vi "HDF5_Write_Noise_Record.vi"(6 "RedundantFileNumber":i32, 7 "LogClust":T1={"base path"=path "C:/Users/Bruce Wayne/Desktop/SourceCode_20171218/thresholds.csv", "PathNow1"=path "", "PathNow2"=path "", "DateNow"="", "NAS path"=path "C:/Users/Bruce Wayne/Desktop/SourceCode_20171218/thresholds.csv", "LogFiltStage"=FALSE, "LogNoise_df_1"=FALSE, "LogNoise_df_2"=FALSE, "LogNoise_df_3"=FALSE, "LogNoise_df_4"=FALSE, "Config"={"UsrCfg"={"Paths"={"CfgFile"=path "", "LogFolder"=path "", "LogFile"=path "", "NAS path"=path "", "ThreshFile"=path "", "RedunFolder"=path ""}, "SampleRate"=12500.0}, "FP_User"={"#NoiseSums"=1, "Max_df"=1, "AvgAvg"=FALSE, "#Avg"=1, "AutoCenter"=FALSE, "Inclin"={"Vmin"=0.0, "Vmax"=0.0, "Angle_min"=0.0, "Angle_max"=0.0, "Offset"=0.0, "Pos_Neg"=FALSE}, "1"={"Cal_"={"Fine"=0.000213623046875, "Coarse_"=4194303.0}, "Beac"={"Fine"=4194303.0, "Coarse_"=1.0}, "Scale"={"Step4"=10000.0, "Step5"=4194303.0, "Step6"=1.0, "Step7"=10000.0}, "Offset"=0.0, "Scale_Noise"=4194303.0, "Scale_Step1"=65535.0, "Scale_In_RT"=1.0, "ScaleMeas"=0.999969482421875, "FreqsToRemove"=[0, 1633], "Width"=[0, 1633], "ScaleMeasEnum"=enum."50", "FilterEnab"=enum."Step 1"}, "2"={"Cal_"={"Fine"=0.000213623046875, "Coarse_"=4194303.0}, "Beac"={"Fine"=0.000213623046875, "Coarse_"=4194303.0}, "Scale"={"Step4"=0.0, "Step5"=4194303.0, "Step6"=1.0, "Step7"=10000.0}, "Offset"=0.0, "Scale_Noise"=4194303.0, "Scale_Step1"=65535.0, "Scale_In_RT"=1.0, "ScaleMeas"=0.999969482421875, "FreqsToRemove"=[0, 1633], "Width"=[0, 1633], "ScaleMeasEnum"=enum."50", "FilterEnab"=enum."Step 1"}, "3"={"Cal_"={"Fine"=0.000213623046875, "Coarse_"=4194303.0}, "Beac"={"Fine"=0.000213623046875, "Coarse_"=4194303.0}, "Scale"={"Step4"=0.0, "Step5"=4194303.0, "Step6"=1.0, "Step7"=10000.0}, "Offset"=0.0, "Scale_Noise"=4194303.0, "Scale_Step1"=65535.0, "Scale_In_RT"=1.0, "ScaleMeas"=0.999969482421875, "FreqsToRemove"=[0, 1633], "Width"=[0, 1633], "ScaleMeasEnum"=enum."50", "FilterEnab"=enum."Step 1"}, "4"={"Cal_"={"Fine"=0.000213623046875, "Coarse_"=4194303.0}, "Beac"={"Fine"=0.000213623046875, "Coarse_"=4194303.0}, "Scale"={"Step4"=0.0, "Step5"=4194303.0, "Step6"=1.0, "Step7"=10000.0}, "Offset"=0.0, "Scale_Noise"=4194303.0, "Scale_Step1"=1.0, "Scale_In_RT"=10000.0, "ScaleMeas"=0.999969482421875, "FreqsToRemove"=[0, 1633], "Width"=[0, 1633], "ScaleMeasEnum"=enum."50", "FilterEnab"=enum."Step 1"}, "Target to Probe"=enum."4", "SNR_Thresh"=1.0, "Paths"={"CfgFile"=path "", "LogFolder"=path "", "LogFile"=path "", "NAS path"=path "", "ThreshFile"=path "", "RedunFolder"=path ""}, "Connex_Location"="", "SimulateFPGA"=FALSE, "Deadband"=0.0}}, "HDFRefs1"={"File"=0, "ToneRefs"=[], "NoiseRefs"=[], "TC_Refs"={"Group_ref"=0, "TimeString_dset"=0, "TimeStamp_dset"=0, "TC0_LP1_Hi"=0, "TC1_LP1_MidHi"=0, "TC2_LP1_Mid"=0, "TC3_LP1_LoMid"=0, "TC4_LP1_Lo"=0, "TC5_LP2_Hi"=0, "TC6_LP2_MidHi"=0, "TC7_LP2_Mid"=0, "TC8_LP2_LoMid"=0, "TC9_LP2_Lo"=0, "TC10_HVAC_Cond_In"=0, "TC11_HVAC_Cond_Out"=0, "TC12_Gen_Exhaust"=0, "TC13_Tamb_Inter"=0}, "ValidRefs"={"Group_ref"=0, "Weath_Valid_dset"=0, "Disdr_Valid_dset"=0, "Saturat_dset"=0, "Alarm_Valid_dset"=0, "Time_Valid_dset"=0, "Time_AlarmChange_dset"=0, "Alarm_Source_dset"=0}, "DisdromRefs"={"BasicGroup_ref"=0, "TimeStamp_dset"=0, "TotalRainRate_dset"=0, "Liquid_dset"=0, "Solid_dset"=0, "TotalRain_dset"=0, "Visibility_dset"=0, "RadarReflect_dset"=0, "MaxDiam_dset"=0, "MeasdParticles_dset"=0, "ParticlMinSpeed_dset"=0, "ParticlMaxSpeed_dset"=0, "ParticlMinDiam_dset"=0, "NonHydrParticls_dset"=0, "NonHydrVolum_dset"=0, "UnknownParticls_dset"=0, "UnknownVolum_dset"=0, "HydromType_dset"=0, "SpectGroup_ref"=0, "Spectrum_dset"=0, "Status_dset_deprecated"=0}, "TE_Refs"={"Group_ref"=0, "TE_Temp1_dset"=0, "TE_Outp1_dset"=0, "TE_Temp2_dset"=0, "TE_Outp2_dset"=0, "TE_Temp3_dset"=0, "TE_Outp3_dset"=0, "TimeStamp"=0}, "UPS_Refs_Deprecated"={"Group_ref"=0, "TimeString_dset"=0, "TimeStamp_dset"=0, "V_dset"=0, "A_dset"=0, "Hz_dset"=0, "W_dset"=0, "%_dset"=0}, "Weath_Refs"={"Group_ref"=0, "TimeString_dset"=0, "TimeStamp_dset "=0, "WindSpd_dset"=0, "WindGusts_dset"=0, "WindDir_dset"=0, "WindDirSTD_dset"=0, "Temp_dset"=0, "Humidity_dset"=0, "Pressure_dset"=0, "RainRate_dset"=0, "RainFall_dset"=0}, "AI_Refs"={"Group_ref"=0, "TimeString_dset"=0, "TimeStamp_dset"=0, "AI0_dset"=0, "AI1_dset"=0, "AI2_dset"=0, "AI3_dset"=0, "AI4_dset"=0, "AI5_dset"=0, "AI6_dset"=0, "AI16_dset"=0, "AI17_dset"=0, "AI18_dset"=0, "AzStdDev_dset"=0, "AI19_dset"=0, "ElStdDev_dset"=0, "BlowerPwr_dset"=0}, "Filter_Refs"={"Filter_Group_ref"=0, "TimeStamp_dset"=0, "Filter_dset"=0}, "ADAM_Refs"={"Group_ref"=0, "ADAM_CoPol_dset"=0, "ADAM_XPol_dset"=0, "ADAM_Noise_dset"=0, "ADAM_CalBox_dset"=0, "TimeStamp"=0}, "Complex"=[]}, "HDFRefs2"={"File"=0, "ToneRefs"=[], "NoiseRefs"=[], "TC_Refs"={"Group_ref"=0, "TimeString_dset"=0, "TimeStamp_dset"=0, "TC0_LP1_Hi"=0, "TC1_LP1_MidHi"=0, "TC2_LP1_Mid"=0, "TC3_LP1_LoMid"=0, "TC4_LP1_Lo"=0, "TC5_LP2_Hi"=0, "TC6_LP2_MidHi"=0, "TC7_LP2_Mid"=0, "TC8_LP2_LoMid"=0, "TC9_LP2_Lo"=0, "TC10_HVAC_Cond_In"=0, "TC11_HVAC_Cond_Out"=0, "TC12_Gen_Exhaust"=0, "TC13_Tamb_Inter"=0}, "ValidRefs"={"Group_ref"=0, "Weath_Valid_dset"=0, "Disdr_Valid_dset"=0, "Saturat_dset"=0, "Alarm_Valid_dset"=0, "Time_Valid_dset"=0, "Time_AlarmChange_dset"=0, "Alarm_Source_dset"=0}, "DisdromRefs"={"BasicGroup_ref"=0, "TimeStamp_dset"=0, "TotalRainRate_dset"=0, "Liquid_dset"=0, "Solid_dset"=0, "TotalRain_dset"=0, "Visibility_dset"=0, "RadarReflect_dset"=0, "MaxDiam_dset"=0, "MeasdParticles_dset"=0, "ParticlMinSpeed_dset"=0, "ParticlMaxSpeed_dset"=0, "ParticlMinDiam_dset"=0, "NonHydrParticls_dset"=0, "NonHydrVolum_dset"=0, "UnknownParticls_dset"=0, "UnknownVolum_dset"=0, "HydromType_dset"=0, "SpectGroup_ref"=0, "Spectrum_dset"=0, "Status_dset_deprecated"=0}, "TE_Refs"={"Group_ref"=0, "TE_Temp1_dset"=0, "TE_Outp1_dset"=0, "TE_Temp2_dset"=0, "TE_Outp2_dset"=0, "TE_Temp3_dset"=0, "TE_Outp3_dset"=0, "TimeStamp"=0}, "UPS_Refs_Deprecated"={"Group_ref"=0, "TimeString_dset"=0, "TimeStamp_dset"=0, "V_dset"=0, "A_dset"=0, "Hz_dset"=0, "W_dset"=0, "%_dset"=0}, "Weath_Refs"={"Group_ref"=0, "TimeString_dset"=0, "TimeStamp_dset "=0, "WindSpd_dset"=0, "WindGusts_dset"=0, "WindDir_dset"=0, "WindDirSTD_dset"=0, "Temp_dset"=0, "Humidity_dset"=0, "Pressure_dset"=0, "RainRate_dset"=0, "RainFall_dset"=0}, "AI_Refs"={"Group_ref"=0, "TimeString_dset"=0, "TimeStamp_dset"=0, "AI0_dset"=0, "AI1_dset"=0, "AI2_dset"=0, "AI3_dset"=0, "AI4_dset"=0, "AI5_dset"=0, "AI6_dset"=0, "AI16_dset"=0, "AI17_dset"=0, "AI18_dset"=0, "AzStdDev_dset"=0, "AI19_dset"=0, "ElStdDev_dset"=0, "BlowerPwr_dset"=0}, "Filter_Refs"={"Filter_Group_ref"=0, "TimeStamp_dset"=0, "Filter_dset"=0}, "ADAM_Refs"={"Group_ref"=0, "ADAM_CoPol_dset"=0, "ADAM_XPol_dset"=0, "ADAM_Noise_dset"=0, "ADAM_CalBox_dset"=0, "TimeStamp"=0}, "Complex"=[]}, "LogData"={"Tone"=[], "TCData"={"TimeStamp"=0.0, "TimeString"="", "TC0_LP1_Hi"=0.0, "TC1_LP1_MidHi"=0.0, "TC2_LP1_Mid"=0.0, "TC3_LP1_LoMid"=0.0, "TC4_LP1_Lo"=0.0, "TC5_LP2_Hi"=0.0, "TC6_LP2_MidHi"=0.0, "TC7_LP2_Mid"=0.0, "TC8_LP2_LoMid"=0.0, "TC9_LP2_Lo"=0.0, "TC10_HVAC_Cond_In"=0.0, "TC11_HVAC_Cond_Out"=0.0, "TC12_Gen_Exhaust"=0.0, "TC13_Amb_Inter"=0.0, "TC14_Unused"=0.0, "TC15_Unused"=0.0, "TC16_Unused"=0.0, "TC17_Unused"=0.0, "TC18_Unused"=0.0, "TC19_Unused"=0.0, "TC20_Unused"=0.0, "TC21_Unused"=0.0, "TC22_Unused"=0.0, "TC23_Unused"=0.0, "TC24_Unused"=0.0, "TC25_Unused"=0.0, "TC26_Unused"=0.0, "TC27_Unused"=0.0, "TC28_Unused"=0.0, "TC29_Unused"=0.0, "TC30_Unused"=0.0, "TC31_Unused"=0.0}, "AI"={"TimeString"="", "Time Stamp"=0.0, "AI0_Unused"=0.0, "AI1_-5V"=0.0, "AI2_+5V"=0.0, "AI3_+6V"=0.0, "AI4_+12V"=0.0, "AI5_+15V"=0.0, "AI6_+28V"=0.0, "AI7_Unused"=0.0, "Ai16_72GHz_CalPower"=0.0, "Ai17_84GHz_CalPower"=0.0, "Ai18_InclinAz"=0.0, "Ai19_InclinEl"=0.0, "Ai20_BlowerPwr"=0.0, "Ai21_Unused"=0.0, "Ai22_Unused"=0.0, "Ai23_Unused"=0.0, "InclinA_StdDev"=0.0, "InclinB_StdDev"=0.0, "InclinAz_Unfilt"=0.0, "InclinEl_Unfilt"=0.0}, "NoiseTrace"=[], "NoiseInfo"=[], "Disdrom"=[], "Weath"=[], "TE"={"TimeString"="", "TimeStamp"=0.0, "Temp"=0.0, "Output"=0.0, "Temp 2"=0.0, "Output 2"=0.0, "Temp 3"=0.0, "Output 3"=0.0}, "ADAM"={"Timestamp"=0.0, "Time string"="", "Fault 1"=FALSE, "Fault 2"=FALSE, "Fault 3"=FALSE, "Fault 4"=FALSE, "Fault 5"=FALSE, "Fault 6"=FALSE, "Value 1"=0.0, "Value 2"=0.0, "Value 3"=0.0, "Value 4"=0.0, "Value 5"=0.0, "Value 6"=0.0}, "TimeDomain"=[]}, "AlarmCfg"={"TC13"={"Enbl"=FALSE, "ErrsAndWarns"={0.0, 5.663716814159292, 7.168141592920354, 8.584070796460177}}, "AI1"={"Enbl"=FALSE, "ErrsAndWarns"={0.0, 5.663716814159292, 7.168141592920354, 8.584070796460177}}, "AI2"={"Enbl"=FALSE, "ErrsAndWarns"={0.0, 5.663716814159292, 7.168141592920354, 8.584070796460177}}, "AI3"={"Enbl"=FALSE, "ErrsAndWarns"={0.0, 5.663716814159292, 7.168141592920354, 8.584070796460177}}, "AI4"={"Enbl"=FALSE, "ErrsAndWarns"={0.0, 5.663716814159292, 7.168141592920354, 8.584070796460177}}, "AI5"={"Enbl"=FALSE, "ErrsAndWarns"={0.0, 5.663716814159292, 7.168141592920354, 8.584070796460177}}, "AI6"={"Enbl"=FALSE, "ErrsAndWarns"={0.0, 5.663716814159292, 7.168141592920354, 8.584070796460177}}, "AI18"={"Enbl"=FALSE, "ErrsAndWarns"={0.0, 5.663716814159292, 7.168141592920354, 8.584070796460177}}, "AI19"={"Enbl"=FALSE, "ErrsAndWarns"={0.0, 5.663716814159292, 7.168141592920354, 8.584070796460177}}, "TE1"={"Enbl"=FALSE, "ErrsAndWarns"={0.0, 5.663716814159292, 7.168141592920354, 8.584070796460177}}, "TE2"={"Enbl"=TRUE, "ErrsAndWarns"={0.0, 5.663716814159292, 7.168141592920354, 8.584070796460177}}, "TE3"={"Enbl"=FALSE, "ErrsAndWarns"={0.0, 5.663716814159292, 7.168141592920354, 8.584070796460177}}, "ADAM1"={"Enbl"=FALSE, "ErrsAndWarns"={0.0, 5.663716814159292, 7.168141592920354, 8.584070796460177}}, "ADAM2"={"Enbl"=FALSE, "ErrsAndWarns"={0.0, 5.663716814159292, 7.168141592920354, 8.584070796460177}}, "ADAM3"={"Enbl"=FALSE, "ErrsAndWarns"={0.0, 5.663716814159292, 7.168141592920354, 8.584070796460177}}, "ADAM4"={"Enbl"=FALSE, "ErrsAndWarns"={0.0, 5.663716814159292, 7.168141592920354, 8.584070796460177}}, "72CoBeacFreq"={"Enbl"=FALSE, "ErrsAndWarns"={0.0, 5.663716814159292, 7.168141592920354, 8.584070796460177}}, "72CoCalFreq"={"Enbl"=FALSE, "ErrsAndWarns"={0.0, 5.663716814159292, 7.168141592920354, 8.584070796460177}}, "84CoBeacFreq"={"Enbl"=FALSE, "ErrsAndWarns"={0.0, 5.663716814159292, 7.168141592920354, 8.584070796460177}}, "84CoCalFreq"={"Enbl"=FALSE, "ErrsAndWarns"={0.0, 5.663716814159292, 7.168141592920354, 8.584070796460177}}, "72Co_CalTonePwr"={"Enbl"=FALSE, "ErrsAndWarns"={0.0, 5.663716814159292, 7.168141592920354, 8.584070796460177}}, "72X_CalTonePwr"={"Enbl"=FALSE, "ErrsAndWarns"={0.0, 5.663716814159292, 7.168141592920354, 8.584070796460177}}, "84Co_CalTonePwr"={"Enbl"=FALSE, "ErrsAndWarns"={0.0, 5.663716814159292, 7.168141592920354, 8.584070796460177}}, "84X_CalTonePwr"={"Enbl"=FALSE, "ErrsAndWarns"={0.0, 5.663716814159292, 7.168141592920354, 8.584070796460177}}}, "DO"=[], "AllAlarms"=[], "Alarm Status"={"Green"=FALSE, "Rx_Yell"=FALSE, "Cx_Yell"=FALSE, "Red"=FALSE, "Source"=""}, "SaturationStatus"={"84"=[], "72"=[]}, "WeatherStatus"=[], "10HzRefs"={"72Co_dset"=0, "84Co_dset"=0, "FileRef"=0}} {"10HzRefs"."FileRef" format="%.0x"; "10HzRefs"."84Co_dset" format="%.0x"; "10HzRefs"."72Co_dset" format="%.0x"; "AlarmCfg"."84X_CalTonePwr"."ErrsAndWarns" scale=-120.0..-45.0; "AlarmCfg"."72X_CalTonePwr"."ErrsAndWarns" scale=-120.0..-45.0; "AlarmCfg"."84Co_CalTonePwr"."ErrsAndWarns" scale=-120.0..-45.0; "AlarmCfg"."72Co_CalTonePwr"."ErrsAndWarns" scale=-120.0..-45.0; "AlarmCfg"."84CoCalFreq"."ErrsAndWarns" scale=24.9..25.1; "AlarmCfg"."84CoBeacFreq"."ErrsAndWarns" scale=25.5..27.0; "AlarmCfg"."72CoCalFreq"."ErrsAndWarns" scale=24.9..25.1; "AlarmCfg"."72CoBeacFreq"."ErrsAndWarns" scale=25.5..27.0; "AlarmCfg"."ADAM4"."ErrsAndWarns" scale=30.0..52.0; "AlarmCfg"."ADAM3"."ErrsAndWarns" scale=30.0..52.0; "AlarmCfg"."ADAM2"."ErrsAndWarns" scale=30.0..52.0; "AlarmCfg"."ADAM1"."ErrsAndWarns" scale=30.0..52.0; "AlarmCfg"."TE3"."ErrsAndWarns" scale=30.0..52.0; "AlarmCfg"."TE2"."ErrsAndWarns" scale=30.0..52.0; "AlarmCfg"."TE1"."ErrsAndWarns" scale=20.0..52.0; "AlarmCfg"."AI19"."ErrsAndWarns" scale=0.0..60.0; "AlarmCfg"."AI18"."ErrsAndWarns" scale=-10.0..10.0; "AlarmCfg"."AI6"."ErrsAndWarns" scale=0.0..35.0; "AlarmCfg"."AI5"."ErrsAndWarns" scale=0.0..20.0; "AlarmCfg"."AI4"."ErrsAndWarns" scale=0.0..15.0; "AlarmCfg"."AI3"."ErrsAndWarns" scale=0.0..10.0; "AlarmCfg"."AI2"."ErrsAndWarns" scale=0.0..10.0; "AlarmCfg"."TC13"."ErrsAndWarns" scale=-10.0..40.0; "LogData"."NoiseInfo"."HDF5_NoiseInfo"."Sum" format="%^#.1g"; "HDFRefs2"."Complex"."Group_ref" format="%.0x"; "HDFRefs2"."Complex"."QSpect_dset" format="%.0x"; "HDFRefs2"."Complex"."ISpect_dset" format="%.0x"; "HDFRefs2"."Complex"."PwrSpect_dset" format="%.0x"; "HDFRefs2"."Complex"."TImeStamp_dset" format="%.0x"; "HDFRefs2"."ADAM_Refs"."Group_ref" format="%.0x"; "HDFRefs2"."ADAM_Refs"."ADAM_CoPol_dset" format="%.0x"; "HDFRefs2"."ADAM_Refs"."ADAM_XPol_dset" format="%.0x"; "HDFRefs2"."ADAM_Refs"."ADAM_Noise_dset" format="%.0x"; "HDFRefs2"."ADAM_Refs"."ADAM_CalBox_dset" format="%.0x"; "HDFRefs2"."ADAM_Refs"."TimeStamp" format="%.0x"; "HDFRefs2"."Filter_Refs"."Filter_Group_ref" format="%.0x"; "HDFRefs2"."Filter_Refs"."TimeStamp_dset" format="%.0x"; "HDFRefs2"."Filter_Refs"."Filter_dset" format="%.0x"; "HDFRefs2"."AI_Refs"."BlowerPwr_dset" format="%.0x"; "HDFRefs2"."AI_Refs"."ElStdDev_dset" format="%.0x"; "HDFRefs2"."AI_Refs"."AzStdDev_dset" format="%.0x"; "HDFRefs2"."AI_Refs"."AI19_dset" format="%.0x"; "HDFRefs2"."AI_Refs"."AI18_dset" format="%.0x"; "HDFRefs2"."AI_Refs"."AI17_dset" format="%.0x"; "HDFRefs2"."AI_Refs"."AI16_dset" format="%.0x"; "HDFRefs2"."AI_Refs"."AI6_dset" format="%.0x"; "HDFRefs2"."AI_Refs"."AI5_dset" format="%.0x"; "HDFRefs2"."AI_Refs"."AI4_dset" format="%.0x"; "HDFRefs2"."AI_Refs"."AI3_dset" format="%.0x"; "HDFRefs2"."AI_Refs"."AI2_dset" format="%.0x"; "HDFRefs2"."AI_Refs"."AI0_dset" format="%.0x"; "HDFRefs2"."AI_Refs"."AI1_dset" format="%.0x"; "HDFRefs2"."AI_Refs"."TimeString_dset" format="%.0x"; "HDFRefs2"."AI_Refs"."TimeStamp_dset" format="%.0x"; "HDFRefs2"."AI_Refs"."Group_ref" format="%.0x"; "HDFRefs2"."Weath_Refs"."WindDirSTD_dset" format="%.0x"; "HDFRefs2"."Weath_Refs"."WindGusts_dset" format="%.0x"; "HDFRefs2"."Weath_Refs"."RainFall_dset" format="%.0x"; "HDFRefs2"."Weath_Refs"."RainRate_dset" format="%.0x"; "HDFRefs2"."Weath_Refs"."Pressure_dset" format="%.0x"; "HDFRefs2"."Weath_Refs"."Humidity_dset" format="%.0x"; "HDFRefs2"."Weath_Refs"."Temp_dset" format="%.0x"; "HDFRefs2"."Weath_Refs"."WindDir_dset" format="%.0x"; "HDFRefs2"."Weath_Refs"."WindSpd_dset" format="%.0x"; "HDFRefs2"."Weath_Refs"."TimeStamp_dset" format="%.0x"; "HDFRefs2"."Weath_Refs"."Group_ref" format="%.0x"; "HDFRefs2"."Weath_Refs"."TimeString_dset" format="%.0x"; "HDFRefs2"."UPS_Refs_Deprecated"."TimeStamp_dset" format="%.0x"; "HDFRefs2"."UPS_Refs_Deprecated"."TimeString_dset" format="%.0x"; "HDFRefs2"."UPS_Refs_Deprecated"."%_dset" format="%.0x"; "HDFRefs2"."UPS_Refs_Deprecated"."W_dset" format="%.0x"; "HDFRefs2"."UPS_Refs_Deprecated"."Hz_dset" format="%.0x"; "HDFRefs2"."UPS_Refs_Deprecated"."A_dset" format="%.0x"; "HDFRefs2"."UPS_Refs_Deprecated"."V_dset" format="%.0x"; "HDFRefs2"."UPS_Refs_Deprecated"."Group_ref" format="%.0x"; "HDFRefs2"."TE_Refs"."TimeStamp" format="%.0x"; "HDFRefs2"."TE_Refs"."TE_Outp3_dset" format="%.0x"; "HDFRefs2"."TE_Refs"."TE_Temp3_dset" format="%.0x"; "HDFRefs2"."TE_Refs"."TE_Outp2_dset" format="%.0x"; "HDFRefs2"."TE_Refs"."TE_Temp2_dset" format="%.0x"; "HDFRefs2"."TE_Refs"."TE_Outp1_dset" format="%.0x"; "HDFRefs2"."TE_Refs"."TE_Temp1_dset" format="%.0x"; "HDFRefs2"."TE_Refs"."Group_ref" format="%.0x"; "HDFRefs2"."DisdromRefs"."Status_dset_deprecated" format="%.0x"; "HDFRefs2"."DisdromRefs"."Spectrum_dset" format="%.0x"; "HDFRefs2"."DisdromRefs"."SpectGroup_ref" format="%.0x"; "HDFRefs2"."DisdromRefs"."HydromType_dset" format="%.0x"; "HDFRefs2"."DisdromRefs"."UnknownVolum_dset" format="%.0x"; "HDFRefs2"."DisdromRefs"."UnknownParticls_dset" format="%.0x"; "HDFRefs2"."DisdromRefs"."NonHydrVolum_dset" format="%.0x"; "HDFRefs2"."DisdromRefs"."NonHydrParticls_dset" format="%.0x"; "HDFRefs2"."DisdromRefs"."ParticlMinDiam_dset" format="%.0x"; "HDFRefs2"."DisdromRefs"."ParticlMaxSpeed_dset" format="%.0x"; "HDFRefs2"."DisdromRefs"."RadarReflect_dset" format="%.0x"; "HDFRefs2"."DisdromRefs"."Visibility_dset" format="%.0x"; "HDFRefs2"."DisdromRefs"."TotalRain_dset" format="%.0x"; "HDFRefs2"."DisdromRefs"."Solid_dset" format="%.0x"; "HDFRefs2"."DisdromRefs"."Liquid_dset" format="%.0x"; "HDFRefs2"."DisdromRefs"."TotalRainRate_dset" format="%.0x"; "HDFRefs2"."DisdromRefs"."TimeStamp_dset" format="%.0x"; "HDFRefs2"."DisdromRefs"."ParticlMinSpeed_dset" format="%.0x"; "HDFRefs2"."DisdromRefs"."MeasdParticles_dset" format="%.0x"; "HDFRefs2"."DisdromRefs"."MaxDiam_dset" format="%.0x"; "HDFRefs2"."DisdromRefs"."BasicGroup_ref" format="%.0x"; "HDFRefs2"."ValidRefs"."Alarm_Source_dset" format="%.0x"; "HDFRefs2"."ValidRefs"."Time_AlarmChange_dset" format="%.0x"; "HDFRefs2"."ValidRefs"."Time_Valid_dset" format="%.0x"; "HDFRefs2"."ValidRefs"."Alarm_Valid_dset" format="%.0x"; "HDFRefs2"."ValidRefs"."Saturat_dset" format="%.0x"; "HDFRefs2"."ValidRefs"."Group_ref" format="%.0x"; "HDFRefs2"."ValidRefs"."Weath_Valid_dset" format="%.0x"; "HDFRefs2"."ValidRefs"."Disdr_Valid_dset" format="%.0x"; "HDFRefs2"."TC_Refs"."TC13_Tamb_Inter" format="%.0x"; "HDFRefs2"."TC_Refs"."TC12_Gen_Exhaust" format="%.0x"; "HDFRefs2"."TC_Refs"."TC11_HVAC_Cond_Out" format="%.0x"; "HDFRefs2"."TC_Refs"."TC10_HVAC_Cond_In" format="%.0x"; "HDFRefs2"."TC_Refs"."TC9_LP2_Lo" format="%.0x"; "HDFRefs2"."TC_Refs"."TC8_LP2_LoMid" format="%.0x"; "HDFRefs2"."TC_Refs"."TC7_LP2_Mid" format="%.0x"; "HDFRefs2"."TC_Refs"."TC6_LP2_MidHi" format="%.0x"; "HDFRefs2"."TC_Refs"."TC5_LP2_Hi" format="%.0x"; "HDFRefs2"."TC_Refs"."TC4_LP1_Lo" format="%.0x"; "HDFRefs2"."TC_Refs"."TC3_LP1_LoMid" format="%.0x"; "HDFRefs2"."TC_Refs"."TC2_LP1_Mid" format="%.0x"; "HDFRefs2"."TC_Refs"."TC1_LP1_MidHi" format="%.0x"; "HDFRefs2"."TC_Refs"."TC0_LP1_Hi" format="%.0x"; "HDFRefs2"."TC_Refs"."TimeString_dset" format="%.0x"; "HDFRefs2"."TC_Refs"."TimeStamp_dset" format="%.0x"; "HDFRefs2"."TC_Refs"."Group_ref" format="%.0x"; "HDFRefs2"."NoiseRefs"."TimeStamp_df_dset" format="%.0x"; "HDFRefs2"."NoiseRefs"."sum_dset" format="%.0x"; "HDFRefs2"."NoiseRefs"."df_dset" format="%.0x"; "HDFRefs2"."NoiseRefs"."TimeStamp_dset" format="%.0x"; "HDFRefs2"."NoiseRefs"."SumdSpectrum_dset" format="%.0x"; "HDFRefs2"."NoiseRefs"."TimeString_dset" format="%.0x"; "HDFRefs2"."NoiseRefs"."Group_ref" format="%.0x"; "HDFRefs2"."ToneRefs"."Group_ref" format="%.0x"; "HDFRefs2"."ToneRefs"."Cal"."Downshift_dset" format="%.0x"; "HDFRefs2"."ToneRefs"."Cal"."DeltaPhase_dset" format="%.0x"; "HDFRefs2"."ToneRefs"."Cal"."Phase_dset" format="%.0x"; "HDFRefs2"."ToneRefs"."Cal"."SNR_dset" format="%.0x"; "HDFRefs2"."ToneRefs"."Cal"."df_dset" format="%.0x"; "HDFRefs2"."ToneRefs"."Cal"."PeakLoc_dset" format="%.0x"; "HDFRefs2"."ToneRefs"."Cal"."MaxValue_dset" format="%.0x"; "HDFRefs2"."ToneRefs"."Cal"."TImeStamp_dset" format="%.0x"; "HDFRefs2"."ToneRefs"."Cal"."TimeString_dset" format="%.0x"; "HDFRefs2"."ToneRefs"."Beac"."Downshift_dset" format="%.0x"; "HDFRefs2"."ToneRefs"."Beac"."DeltaPhase_dset" format="%.0x"; "HDFRefs2"."ToneRefs"."Beac"."Phase_dset" format="%.0x"; "HDFRefs2"."ToneRefs"."Beac"."SNR_dset" format="%.0x"; "HDFRefs2"."ToneRefs"."Beac"."df_dset" format="%.0x"; "HDFRefs2"."ToneRefs"."Beac"."PeakLoc_dset" format="%.0x"; "HDFRefs2"."ToneRefs"."Beac"."MaxValue_dset" format="%.0x"; "HDFRefs2"."ToneRefs"."Beac"."TImeStamp_dset" format="%.0x"; "HDFRefs2"."ToneRefs"."Beac"."TimeString_dset" format="%.0x"; "HDFRefs2"."ToneRefs"."CalZoom_dSet" format="%.0x"; "HDFRefs2"."ToneRefs"."BeacZoom_dSet" format="%.0x"; "HDFRefs2"."File" format="%.0x"; "HDFRefs1"."Complex"."Group_ref" format="%.0x"; "HDFRefs1"."Complex"."QSpect_dset" format="%.0x"; "HDFRefs1"."Complex"."ISpect_dset" format="%.0x"; "HDFRefs1"."Complex"."PwrSpect_dset" format="%.0x"; "HDFRefs1"."Complex"."TImeStamp_dset" format="%.0x"; "HDFRefs1"."ADAM_Refs"."Group_ref" format="%.0x"; "HDFRefs1"."ADAM_Refs"."ADAM_CoPol_dset" format="%.0x"; "HDFRefs1"."ADAM_Refs"."ADAM_XPol_dset" format="%.0x"; "HDFRefs1"."ADAM_Refs"."ADAM_Noise_dset" format="%.0x"; "HDFRefs1"."ADAM_Refs"."ADAM_CalBox_dset" format="%.0x"; "HDFRefs1"."ADAM_Refs"."TimeStamp" format="%.0x"; "HDFRefs1"."Filter_Refs"."Filter_Group_ref" format="%.0x"; "HDFRefs1"."Filter_Refs"."TimeStamp_dset" format="%.0x"; "HDFRefs1"."Filter_Refs"."Filter_dset" format="%.0x"; "HDFRefs1"."AI_Refs"."BlowerPwr_dset" format="%.0x"; "HDFRefs1"."AI_Refs"."ElStdDev_dset" format="%.0x"; "HDFRefs1"."AI_Refs"."AzStdDev_dset" format="%.0x"; "HDFRefs1"."AI_Refs"."AI19_dset" format="%.0x"; "HDFRefs1"."AI_Refs"."AI18_dset" format="%.0x"; "HDFRefs1"."AI_Refs"."AI17_dset" format="%.0x"; "HDFRefs1"."AI_Refs"."AI16_dset" format="%.0x"; "HDFRefs1"."AI_Refs"."AI6_dset" format="%.0x"; "HDFRefs1"."AI_Refs"."AI5_dset" format="%.0x"; "HDFRefs1"."AI_Refs"."AI4_dset" format="%.0x"; "HDFRefs1"."AI_Refs"."AI3_dset" format="%.0x"; "HDFRefs1"."AI_Refs"."AI2_dset" format="%.0x"; "HDFRefs1"."AI_Refs"."AI0_dset" format="%.0x"; "HDFRefs1"."AI_Refs"."AI1_dset" format="%.0x"; "HDFRefs1"."AI_Refs"."TimeString_dset" format="%.0x"; "HDFRefs1"."AI_Refs"."TimeStamp_dset" format="%.0x"; "HDFRefs1"."AI_Refs"."Group_ref" format="%.0x"; "HDFRefs1"."Weath_Refs"."WindDirSTD_dset" format="%.0x"; "HDFRefs1"."Weath_Refs"."WindGusts_dset" format="%.0x"; "HDFRefs1"."Weath_Refs"."RainFall_dset" format="%.0x"; "HDFRefs1"."Weath_Refs"."RainRate_dset" format="%.0x"; "HDFRefs1"."Weath_Refs"."Pressure_dset" format="%.0x"; "HDFRefs1"."Weath_Refs"."Humidity_dset" format="%.0x"; "HDFRefs1"."Weath_Refs"."Temp_dset" format="%.0x"; "HDFRefs1"."Weath_Refs"."WindDir_dset" format="%.0x"; "HDFRefs1"."Weath_Refs"."WindSpd_dset" format="%.0x"; "HDFRefs1"."Weath_Refs"."TimeStamp_dset" format="%.0x"; "HDFRefs1"."Weath_Refs"."Group_ref" format="%.0x"; "HDFRefs1"."Weath_Refs"."TimeString_dset" format="%.0x"; "HDFRefs1"."UPS_Refs_Deprecated"."TimeStamp_dset" format="%.0x"; "HDFRefs1"."UPS_Refs_Deprecated"."TimeString_dset" format="%.0x"; "HDFRefs1"."UPS_Refs_Deprecated"."%_dset" format="%.0x"; "HDFRefs1"."UPS_Refs_Deprecated"."W_dset" format="%.0x"; "HDFRefs1"."UPS_Refs_Deprecated"."Hz_dset" format="%.0x"; "HDFRefs1"."UPS_Refs_Deprecated"."A_dset" format="%.0x"; "HDFRefs1"."UPS_Refs_Deprecated"."V_dset" format="%.0x"; "HDFRefs1"."UPS_Refs_Deprecated"."Group_ref" format="%.0x"; "HDFRefs1"."TE_Refs"."TimeStamp" format="%.0x"; "HDFRefs1"."TE_Refs"."TE_Outp3_dset" format="%.0x"; "HDFRefs1"."TE_Refs"."TE_Temp3_dset" format="%.0x"; "HDFRefs1"."TE_Refs"."TE_Outp2_dset" format="%.0x"; "HDFRefs1"."TE_Refs"."TE_Temp2_dset" format="%.0x"; "HDFRefs1"."TE_Refs"."TE_Outp1_dset" format="%.0x"; "HDFRefs1"."TE_Refs"."TE_Temp1_dset" format="%.0x"; "HDFRefs1"."TE_Refs"."Group_ref" format="%.0x"; "HDFRefs1"."DisdromRefs"."Status_dset_deprecated" format="%.0x"; "HDFRefs1"."DisdromRefs"."Spectrum_dset" format="%.0x"; "HDFRefs1"."DisdromRefs"."SpectGroup_ref" format="%.0x"; "HDFRefs1"."DisdromRefs"."HydromType_dset" format="%.0x"; "HDFRefs1"."DisdromRefs"."UnknownVolum_dset" format="%.0x"; "HDFRefs1"."DisdromRefs"."UnknownParticls_dset" format="%.0x"; "HDFRefs1"."DisdromRefs"."NonHydrVolum_dset" format="%.0x"; "HDFRefs1"."DisdromRefs"."NonHydrParticls_dset" format="%.0x"; "HDFRefs1"."DisdromRefs"."ParticlMinDiam_dset" format="%.0x"; "HDFRefs1"."DisdromRefs"."ParticlMaxSpeed_dset" format="%.0x"; "HDFRefs1"."DisdromRefs"."RadarReflect_dset" format="%.0x"; "HDFRefs1"."DisdromRefs"."Visibility_dset" format="%.0x"; "HDFRefs1"."DisdromRefs"."TotalRain_dset" format="%.0x"; "HDFRefs1"."DisdromRefs"."Solid_dset" format="%.0x"; "HDFRefs1"."DisdromRefs"."Liquid_dset" format="%.0x"; "HDFRefs1"."DisdromRefs"."TotalRainRate_dset" format="%.0x"; "HDFRefs1"."DisdromRefs"."TimeStamp_dset" format="%.0x"; "HDFRefs1"."DisdromRefs"."ParticlMinSpeed_dset" format="%.0x"; "HDFRefs1"."DisdromRefs"."MeasdParticles_dset" format="%.0x"; "HDFRefs1"."DisdromRefs"."MaxDiam_dset" format="%.0x"; "HDFRefs1"."DisdromRefs"."BasicGroup_ref" format="%.0x"; "HDFRefs1"."ValidRefs"."Alarm_Source_dset" format="%.0x"; "HDFRefs1"."ValidRefs"."Time_AlarmChange_dset" format="%.0x"; "HDFRefs1"."ValidRefs"."Time_Valid_dset" format="%.0x"; "HDFRefs1"."ValidRefs"."Alarm_Valid_dset" format="%.0x"; "HDFRefs1"."ValidRefs"."Saturat_dset" format="%.0x"; "HDFRefs1"."ValidRefs"."Group_ref" format="%.0x"; "HDFRefs1"."ValidRefs"."Weath_Valid_dset" format="%.0x"; "HDFRefs1"."ValidRefs"."Disdr_Valid_dset" format="%.0x"; "HDFRefs1"."TC_Refs"."TC13_Tamb_Inter" format="%.0x"; "HDFRefs1"."TC_Refs"."TC12_Gen_Exhaust" format="%.0x"; "HDFRefs1"."TC_Refs"."TC11_HVAC_Cond_Out" format="%.0x"; "HDFRefs1"."TC_Refs"."TC10_HVAC_Cond_In" format="%.0x"; "HDFRefs1"."TC_Refs"."TC9_LP2_Lo" format="%.0x"; "HDFRefs1"."TC_Refs"."TC8_LP2_LoMid" format="%.0x"; "HDFRefs1"."TC_Refs"."TC7_LP2_Mid" format="%.0x"; "HDFRefs1"."TC_Refs"."TC6_LP2_MidHi" format="%.0x"; "HDFRefs1"."TC_Refs"."TC5_LP2_Hi" format="%.0x"; "HDFRefs1"."TC_Refs"."TC4_LP1_Lo" format="%.0x"; "HDFRefs1"."TC_Refs"."TC3_LP1_LoMid" format="%.0x"; "HDFRefs1"."TC_Refs"."TC2_LP1_Mid" format="%.0x"; "HDFRefs1"."TC_Refs"."TC1_LP1_MidHi" format="%.0x"; "HDFRefs1"."TC_Refs"."TC0_LP1_Hi" format="%.0x"; "HDFRefs1"."TC_Refs"."TimeString_dset" format="%.0x"; "HDFRefs1"."TC_Refs"."TimeStamp_dset" format="%.0x"; "HDFRefs1"."TC_Refs"."Group_ref" format="%.0x"; "HDFRefs1"."NoiseRefs"."TimeStamp_df_dset" format="%.0x"; "HDFRefs1"."NoiseRefs"."sum_dset" format="%.0x"; "HDFRefs1"."NoiseRefs"."df_dset" format="%.0x"; "HDFRefs1"."NoiseRefs"."TimeStamp_dset" format="%.0x"; "HDFRefs1"."NoiseRefs"."SumdSpectrum_dset" format="%.0x"; "HDFRefs1"."NoiseRefs"."TimeString_dset" format="%.0x"; "HDFRefs1"."NoiseRefs"."Group_ref" format="%.0x"; "HDFRefs1"."ToneRefs"."Group_ref" format="%.0x"; "HDFRefs1"."ToneRefs"."Cal"."Downshift_dset" format="%.0x"; "HDFRefs1"."ToneRefs"."Cal"."DeltaPhase_dset" format="%.0x"; "HDFRefs1"."ToneRefs"."Cal"."Phase_dset" format="%.0x"; "HDFRefs1"."ToneRefs"."Cal"."SNR_dset" format="%.0x"; "HDFRefs1"."ToneRefs"."Cal"."df_dset" format="%.0x"; "HDFRefs1"."ToneRefs"."Cal"."PeakLoc_dset" format="%.0x"; "HDFRefs1"."ToneRefs"."Cal"."MaxValue_dset" format="%.0x"; "HDFRefs1"."ToneRefs"."Cal"."TImeStamp_dset" format="%.0x"; "HDFRefs1"."ToneRefs"."Cal"."TimeString_dset" format="%.0x"; "HDFRefs1"."ToneRefs"."Beac"."Downshift_dset" format="%.0x"; "HDFRefs1"."ToneRefs"."Beac"."DeltaPhase_dset" format="%.0x"; "HDFRefs1"."ToneRefs"."Beac"."Phase_dset" format="%.0x"; "HDFRefs1"."ToneRefs"."Beac"."SNR_dset" format="%.0x"; "HDFRefs1"."ToneRefs"."Beac"."df_dset" format="%.0x"; "HDFRefs1"."ToneRefs"."Beac"."PeakLoc_dset" format="%.0x"; "HDFRefs1"."ToneRefs"."Beac"."MaxValue_dset" format="%.0x"; "HDFRefs1"."ToneRefs"."Beac"."TImeStamp_dset" format="%.0x"; "HDFRefs1"."ToneRefs"."Beac"."TimeString_dset" format="%.0x"; "HDFRefs1"."ToneRefs"."CalZoom_dSet" format="%.0x"; "HDFRefs1"."ToneRefs"."BeacZoom_dSet" format="%.0x"; "HDFRefs1"."File" format="%.0x"; "Config"."FP_User"."Deadband" format="%#.0f"}, 8 "error in":errorcluster, 9 "HDF5_NoiseInfo":T33={"Timestring"="Timestamp string goes here", "Timestamp"=0.0, "df"=7629.39453125, "Sum"=0.0} {"Sum" format="%^#.1g"}, 10 "Target":T12=enum."4", 11 "NoiseRef":T17 {"TimeStamp_df_dset" format="%.0x"; "sum_dset" format="%.0x"; "df_dset" format="%.0x"; "TimeStamp_dset" format="%.0x"; "SumdSpectrum_dset" format="%.0x"; "TimeString_dset" format="%.0x"; "Group_ref" format="%.0x"}) -> (0 "error out":errorcluster, 5 "LogClust out":T1={"base path"=path "C:/Users/Bruce Wayne/Desktop/SourceCode_20171218/thresholds.csv", "PathNow1"=path "", "PathNow2"=path "", "DateNow"="", "NAS path"=path "C:/Users/Bruce Wayne/Desktop/SourceCode_20171218/thresholds.csv", "LogFiltStage"=FALSE, "LogNoise_df_1"=FALSE, "LogNoise_df_2"=FALSE, "LogNoise_df_3"=FALSE, "LogNoise_df_4"=FALSE, "Config"={"UsrCfg"={"Paths"={"CfgFile"=path "", "LogFolder"=path "", "LogFile"=path "", "NAS path"=path "", "ThreshFile"=path "", "RedunFolder"=path ""}, "SampleRate"=12500.0}, "FP_User"={"#NoiseSums"=1, "Max_df"=1, "AvgAvg"=FALSE, "#Avg"=1, "AutoCenter"=FALSE, "Inclin"={"Vmin"=0.0, "Vmax"=0.0, "Angle_min"=0.0, "Angle_max"=0.0, "Offset"=0.0, "Pos_Neg"=FALSE}, "1"={"Cal_"={"Fine"=0.000213623046875, "Coarse_"=4194303.0}, "Beac"={"Fine"=4194303.0, "Coarse_"=1.0}, "Scale"={"Step4"=10000.0, "Step5"=4194303.0, "Step6"=1.0, "Step7"=10000.0}, "Offset"=0.0, "Scale_Noise"=4194303.0, "Scale_Step1"=65535.0, "Scale_In_RT"=1.0, "ScaleMeas"=0.999969482421875, "FreqsToRemove"=[0, 1633], "Width"=[0, 1633], "ScaleMeasEnum"=enum."50", "FilterEnab"=enum."Step 1"}, "2"={"Cal_"={"Fine"=0.000213623046875, "Coarse_"=4194303.0}, "Beac"={"Fine"=0.000213623046875, "Coarse_"=4194303.0}, "Scale"={"Step4"=0.0, "Step5"=4194303.0, "Step6"=1.0, "Step7"=10000.0}, "Offset"=0.0, "Scale_Noise"=4194303.0, "Scale_Step1"=65535.0, "Scale_In_RT"=1.0, "ScaleMeas"=0.999969482421875, "FreqsToRemove"=[0, 1633], "Width"=[0, 1633], "ScaleMeasEnum"=enum."50", "FilterEnab"=enum."Step 1"}, "3"={"Cal_"={"Fine"=0.000213623046875, "Coarse_"=4194303.0}, "Beac"={"Fine"=0.000213623046875, "Coarse_"=4194303.0}, "Scale"={"Step4"=0.0, "Step5"=4194303.0, "Step6"=1.0, "Step7"=10000.0}, "Offset"=0.0, "Scale_Noise"=4194303.0, "Scale_Step1"=65535.0, "Scale_In_RT"=1.0, "ScaleMeas"=0.999969482421875, "FreqsToRemove"=[0, 1633], "Width"=[0, 1633], "ScaleMeasEnum"=enum."50", "FilterEnab"=enum."Step 1"}, "4"={"Cal_"={"Fine"=0.000213623046875, "Coarse_"=4194303.0}, "Beac"={"Fine"=0.000213623046875, "Coarse_"=4194303.0}, "Scale"={"Step4"=0.0, "Step5"=4194303.0, "Step6"=1.0, "Step7"=10000.0}, "Offset"=0.0, "Scale_Noise"=4194303.0, "Scale_Step1"=1.0, "Scale_In_RT"=10000.0, "ScaleMeas"=0.999969482421875, "FreqsToRemove"=[0, 1633], "Width"=[0, 1633], "ScaleMeasEnum"=enum."50", "FilterEnab"=enum."Step 1"}, "Target to Probe"=enum."4", "SNR_Thresh"=1.0, "Paths"={"CfgFile"=path "", "LogFolder"=path "", "LogFile"=path "", "NAS path"=path "", "ThreshFile"=path "", "RedunFolder"=path ""}, "Connex_Location"="", "SimulateFPGA"=FALSE, "Deadband"=0.0}}, "HDFRefs1"={"File"=0, "ToneRefs"=[], "NoiseRefs"=[], "TC_Refs"={"Group_ref"=0, "TimeString_dset"=0, "TimeStamp_dset"=0, "TC0_LP1_Hi"=0, "TC1_LP1_MidHi"=0, "TC2_LP1_Mid"=0, "TC3_LP1_LoMid"=0, "TC4_LP1_Lo"=0, "TC5_LP2_Hi"=0, "TC6_LP2_MidHi"=0, "TC7_LP2_Mid"=0, "TC8_LP2_LoMid"=0, "TC9_LP2_Lo"=0, "TC10_HVAC_Cond_In"=0, "TC11_HVAC_Cond_Out"=0, "TC12_Gen_Exhaust"=0, "TC13_Tamb_Inter"=0}, "ValidRefs"={"Group_ref"=0, "Weath_Valid_dset"=0, "Disdr_Valid_dset"=0, "Saturat_dset"=0, "Alarm_Valid_dset"=0, "Time_Valid_dset"=0, "Time_AlarmChange_dset"=0, "Alarm_Source_dset"=0}, "DisdromRefs"={"BasicGroup_ref"=0, "TimeStamp_dset"=0, "TotalRainRate_dset"=0, "Liquid_dset"=0, "Solid_dset"=0, "TotalRain_dset"=0, "Visibility_dset"=0, "RadarReflect_dset"=0, "MaxDiam_dset"=0, "MeasdParticles_dset"=0, "ParticlMinSpeed_dset"=0, "ParticlMaxSpeed_dset"=0, "ParticlMinDiam_dset"=0, "NonHydrParticls_dset"=0, "NonHydrVolum_dset"=0, "UnknownParticls_dset"=0, "UnknownVolum_dset"=0, "HydromType_dset"=0, "SpectGroup_ref"=0, "Spectrum_dset"=0, "Status_dset_deprecated"=0}, "TE_Refs"={"Group_ref"=0, "TE_Temp1_dset"=0, "TE_Outp1_dset"=0, "TE_Temp2_dset"=0, "TE_Outp2_dset"=0, "TE_Temp3_dset"=0, "TE_Outp3_dset"=0, "TimeStamp"=0}, "UPS_Refs_Deprecated"={"Group_ref"=0, "TimeString_dset"=0, "TimeStamp_dset"=0, "V_dset"=0, "A_dset"=0, "Hz_dset"=0, "W_dset"=0, "%_dset"=0}, "Weath_Refs"={"Group_ref"=0, "TimeString_dset"=0, "TimeStamp_dset "=0, "WindSpd_dset"=0, "WindGusts_dset"=0, "WindDir_dset"=0, "WindDirSTD_dset"=0, "Temp_dset"=0, "Humidity_dset"=0, "Pressure_dset"=0, "RainRate_dset"=0, "RainFall_dset"=0}, "AI_Refs"={"Group_ref"=0, "TimeString_dset"=0, "TimeStamp_dset"=0, "AI0_dset"=0, "AI1_dset"=0, "AI2_dset"=0, "AI3_dset"=0, "AI4_dset"=0, "AI5_dset"=0, "AI6_dset"=0, "AI16_dset"=0, "AI17_dset"=0, "AI18_dset"=0, "AzStdDev_dset"=0, "AI19_dset"=0, "ElStdDev_dset"=0, "BlowerPwr_dset"=0}, "Filter_Refs"={"Filter_Group_ref"=0, "TimeStamp_dset"=0, "Filter_dset"=0}, "ADAM_Refs"={"Group_ref"=0, "ADAM_CoPol_dset"=0, "ADAM_XPol_dset"=0, "ADAM_Noise_dset"=0, "ADAM_CalBox_dset"=0, "TimeStamp"=0}, "Complex"=[]}, "HDFRefs2"={"File"=0, "ToneRefs"=[], "NoiseRefs"=[], "TC_Refs"={"Group_ref"=0, "TimeString_dset"=0, "TimeStamp_dset"=0, "TC0_LP1_Hi"=0, "TC1_LP1_MidHi"=0, "TC2_LP1_Mid"=0, "TC3_LP1_LoMid"=0, "TC4_LP1_Lo"=0, "TC5_LP2_Hi"=0, "TC6_LP2_MidHi"=0, "TC7_LP2_Mid"=0, "TC8_LP2_LoMid"=0, "TC9_LP2_Lo"=0, "TC10_HVAC_Cond_In"=0, "TC11_HVAC_Cond_Out"=0, "TC12_Gen_Exhaust"=0, "TC13_Tamb_Inter"=0}, "ValidRefs"={"Group_ref"=0, "Weath_Valid_dset"=0, "Disdr_Valid_dset"=0, "Saturat_dset"=0, "Alarm_Valid_dset"=0, "Time_Valid_dset"=0, "Time_AlarmChange_dset"=0, "Alarm_Source_dset"=0}, "DisdromRefs"={"BasicGroup_ref"=0, "TimeStamp_dset"=0, "TotalRainRate_dset"=0, "Liquid_dset"=0, "Solid_dset"=0, "TotalRain_dset"=0, "Visibility_dset"=0, "RadarReflect_dset"=0, "MaxDiam_dset"=0, "MeasdParticles_dset"=0, "ParticlMinSpeed_dset"=0, "ParticlMaxSpeed_dset"=0, "ParticlMinDiam_dset"=0, "NonHydrParticls_dset"=0, "NonHydrVolum_dset"=0, "UnknownParticls_dset"=0, "UnknownVolum_dset"=0, "HydromType_dset"=0, "SpectGroup_ref"=0, "Spectrum_dset"=0, "Status_dset_deprecated"=0}, "TE_Refs"={"Group_ref"=0, "TE_Temp1_dset"=0, "TE_Outp1_dset"=0, "TE_Temp2_dset"=0, "TE_Outp2_dset"=0, "TE_Temp3_dset"=0, "TE_Outp3_dset"=0, "TimeStamp"=0}, "UPS_Refs_Deprecated"={"Group_ref"=0, "TimeString_dset"=0, "TimeStamp_dset"=0, "V_dset"=0, "A_dset"=0, "Hz_dset"=0, "W_dset"=0, "%_dset"=0}, "Weath_Refs"={"Group_ref"=0, "TimeString_dset"=0, "TimeStamp_dset "=0, "WindSpd_dset"=0, "WindGusts_dset"=0, "WindDir_dset"=0, "WindDirSTD_dset"=0, "Temp_dset"=0, "Humidity_dset"=0, "Pressure_dset"=0, "RainRate_dset"=0, "RainFall_dset"=0}, "AI_Refs"={"Group_ref"=0, "TimeString_dset"=0, "TimeStamp_dset"=0, "AI0_dset"=0, "AI1_dset"=0, "AI2_dset"=0, "AI3_dset"=0, "AI4_dset"=0, "AI5_dset"=0, "AI6_dset"=0, "AI16_dset"=0, "AI17_dset"=0, "AI18_dset"=0, "AzStdDev_dset"=0, "AI19_dset"=0, "ElStdDev_dset"=0, "BlowerPwr_dset"=0}, "Filter_Refs"={"Filter_Group_ref"=0, "TimeStamp_dset"=0, "Filter_dset"=0}, "ADAM_Refs"={"Group_ref"=0, "ADAM_CoPol_dset"=0, "ADAM_XPol_dset"=0, "ADAM_Noise_dset"=0, "ADAM_CalBox_dset"=0, "TimeStamp"=0}, "Complex"=[]}, "LogData"={"Tone"=[], "TCData"={"TimeStamp"=0.0, "TimeString"="", "TC0_LP1_Hi"=0.0, "TC1_LP1_MidHi"=0.0, "TC2_LP1_Mid"=0.0, "TC3_LP1_LoMid"=0.0, "TC4_LP1_Lo"=0.0, "TC5_LP2_Hi"=0.0, "TC6_LP2_MidHi"=0.0, "TC7_LP2_Mid"=0.0, "TC8_LP2_LoMid"=0.0, "TC9_LP2_Lo"=0.0, "TC10_HVAC_Cond_In"=0.0, "TC11_HVAC_Cond_Out"=0.0, "TC12_Gen_Exhaust"=0.0, "TC13_Amb_Inter"=0.0, "TC14_Unused"=0.0, "TC15_Unused"=0.0, "TC16_Unused"=0.0, "TC17_Unused"=0.0, "TC18_Unused"=0.0, "TC19_Unused"=0.0, "TC20_Unused"=0.0, "TC21_Unused"=0.0, "TC22_Unused"=0.0, "TC23_Unused"=0.0, "TC24_Unused"=0.0, "TC25_Unused"=0.0, "TC26_Unused"=0.0, "TC27_Unused"=0.0, "TC28_Unused"=0.0, "TC29_Unused"=0.0, "TC30_Unused"=0.0, "TC31_Unused"=0.0}, "AI"={"TimeString"="", "Time Stamp"=0.0, "AI0_Unused"=0.0, "AI1_-5V"=0.0, "AI2_+5V"=0.0, "AI3_+6V"=0.0, "AI4_+12V"=0.0, "AI5_+15V"=0.0, "AI6_+28V"=0.0, "AI7_Unused"=0.0, "Ai16_72GHz_CalPower"=0.0, "Ai17_84GHz_CalPower"=0.0, "Ai18_InclinAz"=0.0, "Ai19_InclinEl"=0.0, "Ai20_BlowerPwr"=0.0, "Ai21_Unused"=0.0, "Ai22_Unused"=0.0, "Ai23_Unused"=0.0, "InclinA_StdDev"=0.0, "InclinB_StdDev"=0.0, "InclinAz_Unfilt"=0.0, "InclinEl_Unfilt"=0.0}, "NoiseTrace"=[], "NoiseInfo"=[], "Disdrom"=[], "Weath"=[], "TE"={"TimeString"="", "TimeStamp"=0.0, "Temp"=0.0, "Output"=0.0, "Temp 2"=0.0, "Output 2"=0.0, "Temp 3"=0.0, "Output 3"=0.0}, "ADAM"={"Timestamp"=0.0, "Time string"="", "Fault 1"=FALSE, "Fault 2"=FALSE, "Fault 3"=FALSE, "Fault 4"=FALSE, "Fault 5"=FALSE, "Fault 6"=FALSE, "Value 1"=0.0, "Value 2"=0.0, "Value 3"=0.0, "Value 4"=0.0, "Value 5"=0.0, "Value 6"=0.0}, "TimeDomain"=[]}, "AlarmCfg"={"TC13"={"Enbl"=FALSE, "ErrsAndWarns"={0.0, 5.663716814159292, 7.168141592920354, 8.584070796460177}}, "AI1"={"Enbl"=FALSE, "ErrsAndWarns"={0.0, 5.663716814159292, 7.168141592920354, 8.584070796460177}}, "AI2"={"Enbl"=FALSE, "ErrsAndWarns"={0.0, 5.663716814159292, 7.168141592920354, 8.584070796460177}}, "AI3"={"Enbl"=FALSE, "ErrsAndWarns"={0.0, 5.663716814159292, 7.168141592920354, 8.584070796460177}}, "AI4"={"Enbl"=FALSE, "ErrsAndWarns"={0.0, 5.663716814159292, 7.168141592920354, 8.584070796460177}}, "AI5"={"Enbl"=FALSE, "ErrsAndWarns"={0.0, 5.663716814159292, 7.168141592920354, 8.584070796460177}}, "AI6"={"Enbl"=FALSE, "ErrsAndWarns"={0.0, 5.663716814159292, 7.168141592920354, 8.584070796460177}}, "AI18"={"Enbl"=FALSE, "ErrsAndWarns"={0.0, 5.663716814159292, 7.168141592920354, 8.584070796460177}}, "AI19"={"Enbl"=FALSE, "ErrsAndWarns"={0.0, 5.663716814159292, 7.168141592920354, 8.584070796460177}}, "TE1"={"Enbl"=FALSE, "ErrsAndWarns"={0.0, 5.663716814159292, 7.168141592920354, 8.584070796460177}}, "TE2"={"Enbl"=TRUE, "ErrsAndWarns"={0.0, 5.663716814159292, 7.168141592920354, 8.584070796460177}}, "TE3"={"Enbl"=FALSE, "ErrsAndWarns"={0.0, 5.663716814159292, 7.168141592920354, 8.584070796460177}}, "ADAM1"={"Enbl"=FALSE, "ErrsAndWarns"={0.0, 5.663716814159292, 7.168141592920354, 8.584070796460177}}, "ADAM2"={"Enbl"=FALSE, "ErrsAndWarns"={0.0, 5.663716814159292, 7.168141592920354, 8.584070796460177}}, "ADAM3"={"Enbl"=FALSE, "ErrsAndWarns"={0.0, 5.663716814159292, 7.168141592920354, 8.584070796460177}}, "ADAM4"={"Enbl"=FALSE, "ErrsAndWarns"={0.0, 5.663716814159292, 7.168141592920354, 8.584070796460177}}, "72CoBeacFreq"={"Enbl"=FALSE, "ErrsAndWarns"={0.0, 5.663716814159292, 7.168141592920354, 8.584070796460177}}, "72CoCalFreq"={"Enbl"=FALSE, "ErrsAndWarns"={0.0, 5.663716814159292, 7.168141592920354, 8.584070796460177}}, "84CoBeacFreq"={"Enbl"=FALSE, "ErrsAndWarns"={0.0, 5.663716814159292, 7.168141592920354, 8.584070796460177}}, "84CoCalFreq"={"Enbl"=FALSE, "ErrsAndWarns"={0.0, 5.663716814159292, 7.168141592920354, 8.584070796460177}}, "72Co_CalTonePwr"={"Enbl"=FALSE, "ErrsAndWarns"={0.0, 5.663716814159292, 7.168141592920354, 8.584070796460177}}, "72X_CalTonePwr"={"Enbl"=FALSE, "ErrsAndWarns"={0.0, 5.663716814159292, 7.168141592920354, 8.584070796460177}}, "84Co_CalTonePwr"={"Enbl"=FALSE, "ErrsAndWarns"={0.0, 5.663716814159292, 7.168141592920354, 8.584070796460177}}, "84X_CalTonePwr"={"Enbl"=FALSE, "ErrsAndWarns"={0.0, 5.663716814159292, 7.168141592920354, 8.584070796460177}}}, "DO"=[], "AllAlarms"=[], "Alarm Status"={"Green"=FALSE, "Rx_Yell"=FALSE, "Cx_Yell"=FALSE, "Red"=FALSE, "Source"=""}, "SaturationStatus"={"84"=[], "72"=[]}, "WeatherStatus"=[], "10HzRefs"={"72Co_dset"=0, "84Co_dset"=0, "FileRef"=0}} {"10HzRefs"."FileRef" format="%.0x"; "10HzRefs"."84Co_dset" format="%.0x"; "10HzRefs"."72Co_dset" format="%.0x"; "AlarmCfg"."84X_CalTonePwr"."ErrsAndWarns" scale=-120.0..-45.0; "AlarmCfg"."72X_CalTonePwr"."ErrsAndWarns" scale=-120.0..-45.0; "AlarmCfg"."84Co_CalTonePwr"."ErrsAndWarns" scale=-120.0..-45.0; "AlarmCfg"."72Co_CalTonePwr"."ErrsAndWarns" scale=-120.0..-45.0; "AlarmCfg"."84CoCalFreq"."ErrsAndWarns" scale=24.9..25.1; "AlarmCfg"."84CoBeacFreq"."ErrsAndWarns" scale=25.5..27.0; "AlarmCfg"."72CoCalFreq"."ErrsAndWarns" scale=24.9..25.1; "AlarmCfg"."72CoBeacFreq"."ErrsAndWarns" scale=25.5..27.0; "AlarmCfg"."ADAM4"."ErrsAndWarns" scale=30.0..52.0; "AlarmCfg"."ADAM3"."ErrsAndWarns" scale=30.0..52.0; "AlarmCfg"."ADAM2"."ErrsAndWarns" scale=30.0..52.0; "AlarmCfg"."ADAM1"."ErrsAndWarns" scale=30.0..52.0; "AlarmCfg"."TE3"."ErrsAndWarns" scale=30.0..52.0; "AlarmCfg"."TE2"."ErrsAndWarns" scale=30.0..52.0; "AlarmCfg"."TE1"."ErrsAndWarns" scale=20.0..52.0; "AlarmCfg"."AI19"."ErrsAndWarns" scale=0.0..60.0; "AlarmCfg"."AI18"."ErrsAndWarns" scale=-10.0..10.0; "AlarmCfg"."AI6"."ErrsAndWarns" scale=0.0..35.0; "AlarmCfg"."AI5"."ErrsAndWarns" scale=0.0..20.0; "AlarmCfg"."AI4"."ErrsAndWarns" scale=0.0..15.0; "AlarmCfg"."AI3"."ErrsAndWarns" scale=0.0..10.0; "AlarmCfg"."AI2"."ErrsAndWarns" scale=0.0..10.0; "AlarmCfg"."TC13"."ErrsAndWarns" scale=-10.0..40.0; "LogData"."NoiseInfo"."HDF5_NoiseInfo"."Sum" format="%^#.1g"; "HDFRefs2"."Complex"."Group_ref" format="%.0x"; "HDFRefs2"."Complex"."QSpect_dset" format="%.0x"; "HDFRefs2"."Complex"."ISpect_dset" format="%.0x"; "HDFRefs2"."Complex"."PwrSpect_dset" format="%.0x"; "HDFRefs2"."Complex"."TImeStamp_dset" format="%.0x"; "HDFRefs2"."ADAM_Refs"."Group_ref" format="%.0x"; "HDFRefs2"."ADAM_Refs"."ADAM_CoPol_dset" format="%.0x"; "HDFRefs2"."ADAM_Refs"."ADAM_XPol_dset" format="%.0x"; "HDFRefs2"."ADAM_Refs"."ADAM_Noise_dset" format="%.0x"; "HDFRefs2"."ADAM_Refs"."ADAM_CalBox_dset" format="%.0x"; "HDFRefs2"."ADAM_Refs"."TimeStamp" format="%.0x"; "HDFRefs2"."Filter_Refs"."Filter_Group_ref" format="%.0x"; "HDFRefs2"."Filter_Refs"."TimeStamp_dset" format="%.0x"; "HDFRefs2"."Filter_Refs"."Filter_dset" format="%.0x"; "HDFRefs2"."AI_Refs"."BlowerPwr_dset" format="%.0x"; "HDFRefs2"."AI_Refs"."ElStdDev_dset" format="%.0x"; "HDFRefs2"."AI_Refs"."AzStdDev_dset" format="%.0x"; "HDFRefs2"."AI_Refs"."AI19_dset" format="%.0x"; "HDFRefs2"."AI_Refs"."AI18_dset" format="%.0x"; "HDFRefs2"."AI_Refs"."AI17_dset" format="%.0x"; "HDFRefs2"."AI_Refs"."AI16_dset" format="%.0x"; "HDFRefs2"."AI_Refs"."AI6_dset" format="%.0x"; "HDFRefs2"."AI_Refs"."AI5_dset" format="%.0x"; "HDFRefs2"."AI_Refs"."AI4_dset" format="%.0x"; "HDFRefs2"."AI_Refs"."AI3_dset" format="%.0x"; "HDFRefs2"."AI_Refs"."AI2_dset" format="%.0x"; "HDFRefs2"."AI_Refs"."AI0_dset" format="%.0x"; "HDFRefs2"."AI_Refs"."AI1_dset" format="%.0x"; "HDFRefs2"."AI_Refs"."TimeString_dset" format="%.0x"; "HDFRefs2"."AI_Refs"."TimeStamp_dset" format="%.0x"; "HDFRefs2"."AI_Refs"."Group_ref" format="%.0x"; "HDFRefs2"."Weath_Refs"."WindDirSTD_dset" format="%.0x"; "HDFRefs2"."Weath_Refs"."WindGusts_dset" format="%.0x"; "HDFRefs2"."Weath_Refs"."RainFall_dset" format="%.0x"; "HDFRefs2"."Weath_Refs"."RainRate_dset" format="%.0x"; "HDFRefs2"."Weath_Refs"."Pressure_dset" format="%.0x"; "HDFRefs2"."Weath_Refs"."Humidity_dset" format="%.0x"; "HDFRefs2"."Weath_Refs"."Temp_dset" format="%.0x"; "HDFRefs2"."Weath_Refs"."WindDir_dset" format="%.0x"; "HDFRefs2"."Weath_Refs"."WindSpd_dset" format="%.0x"; "HDFRefs2"."Weath_Refs"."TimeStamp_dset" format="%.0x"; "HDFRefs2"."Weath_Refs"."Group_ref" format="%.0x"; "HDFRefs2"."Weath_Refs"."TimeString_dset" format="%.0x"; "HDFRefs2"."UPS_Refs_Deprecated"."TimeStamp_dset" format="%.0x"; "HDFRefs2"."UPS_Refs_Deprecated"."TimeString_dset" format="%.0x"; "HDFRefs2"."UPS_Refs_Deprecated"."%_dset" format="%.0x"; "HDFRefs2"."UPS_Refs_Deprecated"."W_dset" format="%.0x"; "HDFRefs2"."UPS_Refs_Deprecated"."Hz_dset" format="%.0x"; "HDFRefs2"."UPS_Refs_Deprecated"."A_dset" format="%.0x"; "HDFRefs2"."UPS_Refs_Deprecated"."V_dset" format="%.0x"; "HDFRefs2"."UPS_Refs_Deprecated"."Group_ref" format="%.0x"; "HDFRefs2"."TE_Refs"."TimeStamp" format="%.0x"; "HDFRefs2"."TE_Refs"."TE_Outp3_dset" format="%.0x"; "HDFRefs2"."TE_Refs"."TE_Temp3_dset" format="%.0x"; "HDFRefs2"."TE_Refs"."TE_Outp2_dset" format="%.0x"; "HDFRefs2"."TE_Refs"."TE_Temp2_dset" format="%.0x"; "HDFRefs2"."TE_Refs"."TE_Outp1_dset" format="%.0x"; "HDFRefs2"."TE_Refs"."TE_Temp1_dset" format="%.0x"; "HDFRefs2"."TE_Refs"."Group_ref" format="%.0x"; "HDFRefs2"."DisdromRefs"."Status_dset_deprecated" format="%.0x"; "HDFRefs2"."DisdromRefs"."Spectrum_dset" format="%.0x"; "HDFRefs2"."DisdromRefs"."SpectGroup_ref" format="%.0x"; "HDFRefs2"."DisdromRefs"."HydromType_dset" format="%.0x"; "HDFRefs2"."DisdromRefs"."UnknownVolum_dset" format="%.0x"; "HDFRefs2"."DisdromRefs"."UnknownParticls_dset" format="%.0x"; "HDFRefs2"."DisdromRefs"."NonHydrVolum_dset" format="%.0x"; "HDFRefs2"."DisdromRefs"."NonHydrParticls_dset" format="%.0x"; "HDFRefs2"."DisdromRefs"."ParticlMinDiam_dset" format="%.0x"; "HDFRefs2"."DisdromRefs"."ParticlMaxSpeed_dset" format="%.0x"; "HDFRefs2"."DisdromRefs"."RadarReflect_dset" format="%.0x"; "HDFRefs2"."DisdromRefs"."Visibility_dset" format="%.0x"; "HDFRefs2"."DisdromRefs"."TotalRain_dset" format="%.0x"; "HDFRefs2"."DisdromRefs"."Solid_dset" format="%.0x"; "HDFRefs2"."DisdromRefs"."Liquid_dset" format="%.0x"; "HDFRefs2"."DisdromRefs"."TotalRainRate_dset" format="%.0x"; "HDFRefs2"."DisdromRefs"."TimeStamp_dset" format="%.0x"; "HDFRefs2"."DisdromRefs"."ParticlMinSpeed_dset" format="%.0x"; "HDFRefs2"."DisdromRefs"."MeasdParticles_dset" format="%.0x"; "HDFRefs2"."DisdromRefs"."MaxDiam_dset" format="%.0x"; "HDFRefs2"."DisdromRefs"."BasicGroup_ref" format="%.0x"; "HDFRefs2"."ValidRefs"."Alarm_Source_dset" format="%.0x"; "HDFRefs2"."ValidRefs"."Time_AlarmChange_dset" format="%.0x"; "HDFRefs2"."ValidRefs"."Time_Valid_dset" format="%.0x"; "HDFRefs2"."ValidRefs"."Alarm_Valid_dset" format="%.0x"; "HDFRefs2"."ValidRefs"."Saturat_dset" format="%.0x"; "HDFRefs2"."ValidRefs"."Group_ref" format="%.0x"; "HDFRefs2"."ValidRefs"."Weath_Valid_dset" format="%.0x"; "HDFRefs2"."ValidRefs"."Disdr_Valid_dset" format="%.0x"; "HDFRefs2"."TC_Refs"."TC13_Tamb_Inter" format="%.0x"; "HDFRefs2"."TC_Refs"."TC12_Gen_Exhaust" format="%.0x"; "HDFRefs2"."TC_Refs"."TC11_HVAC_Cond_Out" format="%.0x"; "HDFRefs2"."TC_Refs"."TC10_HVAC_Cond_In" format="%.0x"; "HDFRefs2"."TC_Refs"."TC9_LP2_Lo" format="%.0x"; "HDFRefs2"."TC_Refs"."TC8_LP2_LoMid" format="%.0x"; "HDFRefs2"."TC_Refs"."TC7_LP2_Mid" format="%.0x"; "HDFRefs2"."TC_Refs"."TC6_LP2_MidHi" format="%.0x"; "HDFRefs2"."TC_Refs"."TC5_LP2_Hi" format="%.0x"; "HDFRefs2"."TC_Refs"."TC4_LP1_Lo" format="%.0x"; "HDFRefs2"."TC_Refs"."TC3_LP1_LoMid" format="%.0x"; "HDFRefs2"."TC_Refs"."TC2_LP1_Mid" format="%.0x"; "HDFRefs2"."TC_Refs"."TC1_LP1_MidHi" format="%.0x"; "HDFRefs2"."TC_Refs"."TC0_LP1_Hi" format="%.0x"; "HDFRefs2"."TC_Refs"."TimeString_dset" format="%.0x"; "HDFRefs2"."TC_Refs"."TimeStamp_dset" format="%.0x"; "HDFRefs2"."TC_Refs"."Group_ref" format="%.0x"; "HDFRefs2"."NoiseRefs"."TimeStamp_df_dset" format="%.0x"; "HDFRefs2"."NoiseRefs"."sum_dset" format="%.0x"; "HDFRefs2"."NoiseRefs"."df_dset" format="%.0x"; "HDFRefs2"."NoiseRefs"."TimeStamp_dset" format="%.0x"; "HDFRefs2"."NoiseRefs"."SumdSpectrum_dset" format="%.0x"; "HDFRefs2"."NoiseRefs"."TimeString_dset" format="%.0x"; "HDFRefs2"."NoiseRefs"."Group_ref" format="%.0x"; "HDFRefs2"."ToneRefs"."Group_ref" format="%.0x"; "HDFRefs2"."ToneRefs"."Cal"."Downshift_dset" format="%.0x"; "HDFRefs2"."ToneRefs"."Cal"."DeltaPhase_dset" format="%.0x"; "HDFRefs2"."ToneRefs"."Cal"."Phase_dset" format="%.0x"; "HDFRefs2"."ToneRefs"."Cal"."SNR_dset" format="%.0x"; "HDFRefs2"."ToneRefs"."Cal"."df_dset" format="%.0x"; "HDFRefs2"."ToneRefs"."Cal"."PeakLoc_dset" format="%.0x"; "HDFRefs2"."ToneRefs"."Cal"."MaxValue_dset" format="%.0x"; "HDFRefs2"."ToneRefs"."Cal"."TImeStamp_dset" format="%.0x"; "HDFRefs2"."ToneRefs"."Cal"."TimeString_dset" format="%.0x"; "HDFRefs2"."ToneRefs"."Beac"."Downshift_dset" format="%.0x"; "HDFRefs2"."ToneRefs"."Beac"."DeltaPhase_dset" format="%.0x"; "HDFRefs2"."ToneRefs"."Beac"."Phase_dset" format="%.0x"; "HDFRefs2"."ToneRefs"."Beac"."SNR_dset" format="%.0x"; "HDFRefs2"."ToneRefs"."Beac"."df_dset" format="%.0x"; "HDFRefs2"."ToneRefs"."Beac"."PeakLoc_dset" format="%.0x"; "HDFRefs2"."ToneRefs"."Beac"."MaxValue_dset" format="%.0x"; "HDFRefs2"."ToneRefs"."Beac"."TImeStamp_dset" format="%.0x"; "HDFRefs2"."ToneRefs"."Beac"."TimeString_dset" format="%.0x"; "HDFRefs2"."ToneRefs"."CalZoom_dSet" format="%.0x"; "HDFRefs2"."ToneRefs"."BeacZoom_dSet" format="%.0x"; "HDFRefs2"."File" format="%.0x"; "HDFRefs1"."Complex"."Group_ref" format="%.0x"; "HDFRefs1"."Complex"."QSpect_dset" format="%.0x"; "HDFRefs1"."Complex"."ISpect_dset" format="%.0x"; "HDFRefs1"."Complex"."PwrSpect_dset" format="%.0x"; "HDFRefs1"."Complex"."TImeStamp_dset" format="%.0x"; "HDFRefs1"."ADAM_Refs"."Group_ref" format="%.0x"; "HDFRefs1"."ADAM_Refs"."ADAM_CoPol_dset" format="%.0x"; "HDFRefs1"."ADAM_Refs"."ADAM_XPol_dset" format="%.0x"; "HDFRefs1"."ADAM_Refs"."ADAM_Noise_dset" format="%.0x"; "HDFRefs1"."ADAM_Refs"."ADAM_CalBox_dset" format="%.0x"; "HDFRefs1"."ADAM_Refs"."TimeStamp" format="%.0x"; "HDFRefs1"."Filter_Refs"."Filter_Group_ref" format="%.0x"; "HDFRefs1"."Filter_Refs"."TimeStamp_dset" format="%.0x"; "HDFRefs1"."Filter_Refs"."Filter_dset" format="%.0x"; "HDFRefs1"."AI_Refs"."BlowerPwr_dset" format="%.0x"; "HDFRefs1"."AI_Refs"."ElStdDev_dset" format="%.0x"; "HDFRefs1"."AI_Refs"."AzStdDev_dset" format="%.0x"; "HDFRefs1"."AI_Refs"."AI19_dset" format="%.0x"; "HDFRefs1"."AI_Refs"."AI18_dset" format="%.0x"; "HDFRefs1"."AI_Refs"."AI17_dset" format="%.0x"; "HDFRefs1"."AI_Refs"."AI16_dset" format="%.0x"; "HDFRefs1"."AI_Refs"."AI6_dset" format="%.0x"; "HDFRefs1"."AI_Refs"."AI5_dset" format="%.0x"; "HDFRefs1"."AI_Refs"."AI4_dset" format="%.0x"; "HDFRefs1"."AI_Refs"."AI3_dset" format="%.0x"; "HDFRefs1"."AI_Refs"."AI2_dset" format="%.0x"; "HDFRefs1"."AI_Refs"."AI0_dset" format="%.0x"; "HDFRefs1"."AI_Refs"."AI1_dset" format="%.0x"; "HDFRefs1"."AI_Refs"."TimeString_dset" format="%.0x"; "HDFRefs1"."AI_Refs"."TimeStamp_dset" format="%.0x"; "HDFRefs1"."AI_Refs"."Group_ref" format="%.0x"; "HDFRefs1"."Weath_Refs"."WindDirSTD_dset" format="%.0x"; "HDFRefs1"."Weath_Refs"."WindGusts_dset" format="%.0x"; "HDFRefs1"."Weath_Refs"."RainFall_dset" format="%.0x"; "HDFRefs1"."Weath_Refs"."RainRate_dset" format="%.0x"; "HDFRefs1"."Weath_Refs"."Pressure_dset" format="%.0x"; "HDFRefs1"."Weath_Refs"."Humidity_dset" format="%.0x"; "HDFRefs1"."Weath_Refs"."Temp_dset" format="%.0x"; "HDFRefs1"."Weath_Refs"."WindDir_dset" format="%.0x"; "HDFRefs1"."Weath_Refs"."WindSpd_dset" format="%.0x"; "HDFRefs1"."Weath_Refs"."TimeStamp_dset" format="%.0x"; "HDFRefs1"."Weath_Refs"."Group_ref" format="%.0x"; "HDFRefs1"."Weath_Refs"."TimeString_dset" format="%.0x"; "HDFRefs1"."UPS_Refs_Deprecated"."TimeStamp_dset" format="%.0x"; "HDFRefs1"."UPS_Refs_Deprecated"."TimeString_dset" format="%.0x"; "HDFRefs1"."UPS_Refs_Deprecated"."%_dset" format="%.0x"; "HDFRefs1"."UPS_Refs_Deprecated"."W_dset" format="%.0x"; "HDFRefs1"."UPS_Refs_Deprecated"."Hz_dset" format="%.0x"; "HDFRefs1"."UPS_Refs_Deprecated"."A_dset" format="%.0x"; "HDFRefs1"."UPS_Refs_Deprecated"."V_dset" format="%.0x"; "HDFRefs1"."UPS_Refs_Deprecated"."Group_ref" format="%.0x"; "HDFRefs1"."TE_Refs"."TimeStamp" format="%.0x"; "HDFRefs1"."TE_Refs"."TE_Outp3_dset" format="%.0x"; "HDFRefs1"."TE_Refs"."TE_Temp3_dset" format="%.0x"; "HDFRefs1"."TE_Refs"."TE_Outp2_dset" format="%.0x"; "HDFRefs1"."TE_Refs"."TE_Temp2_dset" format="%.0x"; "HDFRefs1"."TE_Refs"."TE_Outp1_dset" format="%.0x"; "HDFRefs1"."TE_Refs"."TE_Temp1_dset" format="%.0x"; "HDFRefs1"."TE_Refs"."Group_ref" format="%.0x"; "HDFRefs1"."DisdromRefs"."Status_dset_deprecated" format="%.0x"; "HDFRefs1"."DisdromRefs"."Spectrum_dset" format="%.0x"; "HDFRefs1"."DisdromRefs"."SpectGroup_ref" format="%.0x"; "HDFRefs1"."DisdromRefs"."HydromType_dset" format="%.0x"; "HDFRefs1"."DisdromRefs"."UnknownVolum_dset" format="%.0x"; "HDFRefs1"."DisdromRefs"."UnknownParticls_dset" format="%.0x"; "HDFRefs1"."DisdromRefs"."NonHydrVolum_dset" format="%.0x"; "HDFRefs1"."DisdromRefs"."NonHydrParticls_dset" format="%.0x"; "HDFRefs1"."DisdromRefs"."ParticlMinDiam_dset" format="%.0x"; "HDFRefs1"."DisdromRefs"."ParticlMaxSpeed_dset" format="%.0x"; "HDFRefs1"."DisdromRefs"."RadarReflect_dset" format="%.0x"; "HDFRefs1"."DisdromRefs"."Visibility_dset" format="%.0x"; "HDFRefs1"."DisdromRefs"."TotalRain_dset" format="%.0x"; "HDFRefs1"."DisdromRefs"."Solid_dset" format="%.0x"; "HDFRefs1"."DisdromRefs"."Liquid_dset" format="%.0x"; "HDFRefs1"."DisdromRefs"."TotalRainRate_dset" format="%.0x"; "HDFRefs1"."DisdromRefs"."TimeStamp_dset" format="%.0x"; "HDFRefs1"."DisdromRefs"."ParticlMinSpeed_dset" format="%.0x"; "HDFRefs1"."DisdromRefs"."MeasdParticles_dset" format="%.0x"; "HDFRefs1"."DisdromRefs"."MaxDiam_dset" format="%.0x"; "HDFRefs1"."DisdromRefs"."BasicGroup_ref" format="%.0x"; "HDFRefs1"."ValidRefs"."Alarm_Source_dset" format="%.0x"; "HDFRefs1"."ValidRefs"."Time_AlarmChange_dset" format="%.0x"; "HDFRefs1"."ValidRefs"."Time_Valid_dset" format="%.0x"; "HDFRefs1"."ValidRefs"."Alarm_Valid_dset" format="%.0x"; "HDFRefs1"."ValidRefs"."Saturat_dset" format="%.0x"; "HDFRefs1"."ValidRefs"."Group_ref" format="%.0x"; "HDFRefs1"."ValidRefs"."Weath_Valid_dset" format="%.0x"; "HDFRefs1"."ValidRefs"."Disdr_Valid_dset" format="%.0x"; "HDFRefs1"."TC_Refs"."TC13_Tamb_Inter" format="%.0x"; "HDFRefs1"."TC_Refs"."TC12_Gen_Exhaust" format="%.0x"; "HDFRefs1"."TC_Refs"."TC11_HVAC_Cond_Out" format="%.0x"; "HDFRefs1"."TC_Refs"."TC10_HVAC_Cond_In" format="%.0x"; "HDFRefs1"."TC_Refs"."TC9_LP2_Lo" format="%.0x"; "HDFRefs1"."TC_Refs"."TC8_LP2_LoMid" format="%.0x"; "HDFRefs1"."TC_Refs"."TC7_LP2_Mid" format="%.0x"; "HDFRefs1"."TC_Refs"."TC6_LP2_MidHi" format="%.0x"; "HDFRefs1"."TC_Refs"."TC5_LP2_Hi" format="%.0x"; "HDFRefs1"."TC_Refs"."TC4_LP1_Lo" format="%.0x"; "HDFRefs1"."TC_Refs"."TC3_LP1_LoMid" format="%.0x"; "HDFRefs1"."TC_Refs"."TC2_LP1_Mid" format="%.0x"; "HDFRefs1"."TC_Refs"."TC1_LP1_MidHi" format="%.0x"; "HDFRefs1"."TC_Refs"."TC0_LP1_Hi" format="%.0x"; "HDFRefs1"."TC_Refs"."TimeString_dset" format="%.0x"; "HDFRefs1"."TC_Refs"."TimeStamp_dset" format="%.0x"; "HDFRefs1"."TC_Refs"."Group_ref" format="%.0x"; "HDFRefs1"."NoiseRefs"."TimeStamp_df_dset" format="%.0x"; "HDFRefs1"."NoiseRefs"."sum_dset" format="%.0x"; "HDFRefs1"."NoiseRefs"."df_dset" format="%.0x"; "HDFRefs1"."NoiseRefs"."TimeStamp_dset" format="%.0x"; "HDFRefs1"."NoiseRefs"."SumdSpectrum_dset" format="%.0x"; "HDFRefs1"."NoiseRefs"."TimeString_dset" format="%.0x"; "HDFRefs1"."NoiseRefs"."Group_ref" format="%.0x"; "HDFRefs1"."ToneRefs"."Group_ref" format="%.0x"; "HDFRefs1"."ToneRefs"."Cal"."Downshift_dset" format="%.0x"; "HDFRefs1"."ToneRefs"."Cal"."DeltaPhase_dset" format="%.0x"; "HDFRefs1"."ToneRefs"."Cal"."Phase_dset" format="%.0x"; "HDFRefs1"."ToneRefs"."Cal"."SNR_dset" format="%.0x"; "HDFRefs1"."ToneRefs"."Cal"."df_dset" format="%.0x"; "HDFRefs1"."ToneRefs"."Cal"."PeakLoc_dset" format="%.0x"; "HDFRefs1"."ToneRefs"."Cal"."MaxValue_dset" format="%.0x"; "HDFRefs1"."ToneRefs"."Cal"."TImeStamp_dset" format="%.0x"; "HDFRefs1"."ToneRefs"."Cal"."TimeString_dset" format="%.0x"; "HDFRefs1"."ToneRefs"."Beac"."Downshift_dset" format="%.0x"; "HDFRefs1"."ToneRefs"."Beac"."DeltaPhase_dset" format="%.0x"; "HDFRefs1"."ToneRefs"."Beac"."Phase_dset" format="%.0x"; "HDFRefs1"."ToneRefs"."Beac"."SNR_dset" format="%.0x"; "HDFRefs1"."ToneRefs"."Beac"."df_dset" format="%.0x"; "HDFRefs1"."ToneRefs"."Beac"."PeakLoc_dset" format="%.0x"; "HDFRefs1"."ToneRefs"."Beac"."MaxValue_dset" format="%.0x"; "HDFRefs1"."ToneRefs"."Beac"."TImeStamp_dset" format="%.0x"; "HDFRefs1"."ToneRefs"."Beac"."TimeString_dset" format="%.0x"; "HDFRefs1"."ToneRefs"."CalZoom_dSet" format="%.0x"; "HDFRefs1"."ToneRefs"."BeacZoom_dSet" format="%.0x"; "HDFRefs1"."File" format="%.0x"; "Config"."FP_User"."Deadband" format="%#.0f"})   [LabVIEW 2018]
doc: "Write a single Noise<x> record with timestamp:\nNoise1\n NoiseInfo - cluster with Timestamp and other metadata for this record\n SummdSpectrum - 1024 element Double array (waveform)"
uses:
  HDF5_Noise_refs.ctl
  <vilib>/addons/h5labview2/base/hid_t.ctl
  HDF5_NoiseInfoClust.ctl
  Controls/Clusts/LogLoopClust.ctl
  Controls/Clusts/Config_Clust.ctl
  Controls/Clusts/UserConfig.ctl
  Controls/PathsCluster.ctl
  Controls/Clusts/FrontPanel_UserConfig.ctl
  Controls/Clusts/Inclinometer_User_Cfg.ctl
  Controls/Clusts/FP_UserTargetConfig.ctl
  Controls/Clusts/FreqShift.ctl
  Controls/Clusts/FPGA_Scale.ctl
  Controls/Enums/ScaleMeasure.ctl
  Controls/RadioButtons/FilterEnableRadio.ctl
  Controls/Enums/TargetNumber.ctl
  Controls/Clusts/HDF5_File_Refs.ctl
  Controls/Clusts/ToneGroupRefsClust.ctl
  HDF5_Tone_refs.ctl
  TC_Tone_refs.ctl
  HDF5_Validty_refs.ctl
  HDF5_Disdrometer_Refs.ctl
  HDF5_Health_Refs.ctl
  UPS_refs.ctl
  Controls/Clusts/WeatherRefs.ctl
  HDF5_AI_refs.ctl
  HDF5_Filter_refs.ctl
  HDF5_ADAM_Refs.ctl
  HDF5_Complex_Refs.ctl
  Controls/Clusts/LogDataClust.ctl
  Controls/Clusts/ToneLogBuffered.ctl
  Controls/Clusts/SaturationMonitorBuffer.ctl
  TC_Data_Structure.ctl
  Controls/Clusts/AI_Clust.ctl
  DisdrometerData.ctl
  DisdromterSummaryData.ctl
  Disdrometer/Disdrometer_Status_Cluster.ctl
  Controls/Clusts/WeatherDataClust.ctl
  Controls/Clusts/ValidityWeatherClust.ctl
  Controls/Clusts/TE_Data_Clust.ctl
  HDF5_ADAM_Data.ctl
  Controls/Clusts/TimeDomainData.ctl
  Controls/Clusts/AlarmSettingsClust.ctl
  Controls/Clusts/AlarmThresh_OneChan.ctl
  Controls/Clusts/ErrorStatus.ctl
  Controls/Clusts/DigOutClust.ctl
  Controls/Clusts/Saturation_Status_Clust.ctl
  Controls/Clusts/HDF5_10HzRefs.ctl
  <vilib>/addons/h5labview2/base/lib_path.vi
  <vilib>/addons/h5labview2/base/H5Equery.vi
  lib_path_mod_20200519.vi
  <vilib>/addons/h5labview2/dataset/H5Dwrite.llb/H5Dwrite.xnode
  <vilib>/addons/h5labview2/dataset/H5D.lvlib
  <vilib>/addons/h5labview2/space/H5S.lvlib
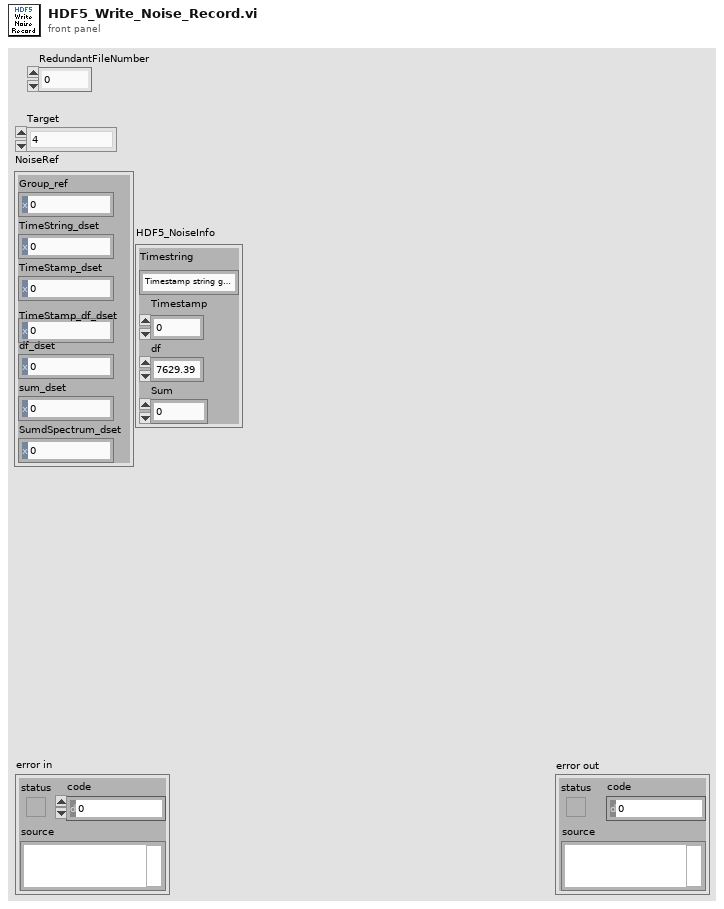
[diagram p1: front panel]
types:
  T1 = typedef "LogLoopClust.ctl" = cluster{"base path":path, "PathNow1":path, "PathNow2":path, "DateNow":string, "NAS path":path, "LogFiltStage":bool, "LogNoise_df_1":bool, "LogNoise_df_2":bool, "LogNoise_df_3":bool, "LogNoise_df_4":bool, "Config":T2, "HDFRefs1":T13, "HDFRefs2":T13, "LogData":T28, "AlarmCfg":T42, "DO":bool[], "AllAlarms":T44[], "Alarm Status":T45, "SaturationStatus":T46, "WeatherStatus":bool[], "10HzRefs":T47}
  T2 = typedef "Config_Clust.ctl" = cluster{"UsrCfg":T3, "FP_User":T5}
  T3 = typedef "UserConfig.ctl" = cluster{"Paths":T4, "SampleRate":dbl}
  T4 = typedef "PathsCluster.ctl" = cluster{"CfgFile":path, "LogFolder":path, "LogFile":path, "NAS path":path, "ThreshFile":path, "RedunFolder":path}
  T5 = typedef "FrontPanel_UserConfig.ctl" = cluster{"#NoiseSums":u32, "Max_df":u32, "AvgAvg":bool, "#Avg":u16, "AutoCenter":bool, "Inclin":T6, "1":T7, "2":T7, "3":T7, "4":T7, "Target to Probe":T12, "SNR_Thresh":dbl, "Paths":T4, "Connex_Location":string, "SimulateFPGA":bool, "Deadband":dbl}
  T6 = typedef "Inclinometer_User_Cfg.ctl" = cluster{"Vmin":dbl, "Vmax":dbl, "Angle_min":dbl, "Angle_max":dbl, "Offset":dbl, "Pos_Neg":bool}
  T7 = typedef "FP_UserTargetConfig.ctl" = cluster{"Cal_":T8, "Beac":T8, "Scale":T9, "Offset":fxp<+/-,16,16>, "Scale_Noise":fxp<+/-,30,30>, "Scale_Step1":fxp<+/-,17,17>, "Scale_In_RT":ext, "ScaleMeas":fxp<+/-,16,1>, "FreqsToRemove":i32[], "Width":i32[], "ScaleMeasEnum":T10, "FilterEnab":T11}
  T8 = typedef "FreqShift.ctl" = cluster{"Fine":dbl, "Coarse_":dbl}
  T9 = typedef "FPGA_Scale.ctl" = cluster{"Step4":fxp<+/-,23,23>, "Step5":fxp<+/-,23,23>, "Step6":fxp<+/-,23,23>, "Step7":fxp<+/-,23,23>}
  T10 = typedef "ScaleMeasure.ctl" = enum16{"1", "10", "50", "42"}
  T11 = typedef "FilterEnableRadio.ctl" = enum32{"None", "Step 1", "Frequency Shift", "Step 4", "Step 5", "Step 6", "Step 7"}
  T12 = typedef "TargetNumber.ctl" = enum16{"1", "2", "3", "4"}
  T13 = typedef "HDF5_File_Refs.ctl" = cluster{"File":T14, "ToneRefs":T15[], "NoiseRefs":T17[], "TC_Refs":T18, "ValidRefs":T19, "DisdromRefs":T20, "TE_Refs":T21, "UPS_Refs_Deprecated":T22, "Weath_Refs":T23, "AI_Refs":T24, "Filter_Refs":T25, "ADAM_Refs":T26, "Complex":T27[]}
  T14 = typedef "hid_t.ctl" = i32
  T15 = typedef "ToneGroupRefsClust.ctl" = cluster{"Group_ref":T14, "Cal":T16, "Beac":T16, "CalZoom_dSet":T14, "BeacZoom_dSet":T14}
  T16 = typedef "HDF5_Tone_refs.ctl" = cluster{"TimeString_dset":T14, "TImeStamp_dset":T14, "SNR_dset":T14, "MaxValue_dset":T14, "PeakLoc_dset":T14, "df_dset":T14, "Phase_dset":T14, "DeltaPhase_dset":T14, "Downshift_dset":T14}
  T17 = typedef "HDF5_Noise_refs.ctl" = cluster{"Group_ref":T14, "TimeString_dset":T14, "TimeStamp_dset":T14, "TimeStamp_df_dset":T14, "df_dset":T14, "sum_dset":T14, "SumdSpectrum_dset":T14}
  T18 = typedef "TC_Tone_refs.ctl" = cluster{"Group_ref":T14, "TimeString_dset":T14, "TimeStamp_dset":T14, "TC0_LP1_Hi":T14, "TC1_LP1_MidHi":T14, "TC2_LP1_Mid":T14, "TC3_LP1_LoMid":T14, "TC4_LP1_Lo":T14, "TC5_LP2_Hi":T14, "TC6_LP2_MidHi":T14, "TC7_LP2_Mid":T14, "TC8_LP2_LoMid":T14, "TC9_LP2_Lo":T14, "TC10_HVAC_Cond_In":T14, "TC11_HVAC_Cond_Out":T14, "TC12_Gen_Exhaust":T14, "TC13_Tamb_Inter":T14}
  T19 = typedef "HDF5_Validty_refs.ctl" = cluster{"Group_ref":T14, "Weath_Valid_dset":T14, "Disdr_Valid_dset":T14, "Saturat_dset":T14, "Alarm_Valid_dset":T14, "Time_Valid_dset":T14, "Time_AlarmChange_dset":T14, "Alarm_Source_dset":T14}
  T20 = typedef "HDF5_Disdrometer_Refs.ctl" = cluster{"BasicGroup_ref":T14, "TimeStamp_dset":T14, "TotalRainRate_dset":T14, "Liquid_dset":T14, "Solid_dset":T14, "TotalRain_dset":T14, "Visibility_dset":T14, "RadarReflect_dset":T14, "MaxDiam_dset":T14, "MeasdParticles_dset":T14, "ParticlMinSpeed_dset":T14, "ParticlMaxSpeed_dset":T14, "ParticlMinDiam_dset":T14, "NonHydrParticls_dset":T14, "NonHydrVolum_dset":T14, "UnknownParticls_dset":T14, "UnknownVolum_dset":T14, "HydromType_dset":T14, "SpectGroup_ref":T14, "Spectrum_dset":T14, "Status_dset_deprecated":T14}
  T21 = typedef "HDF5_Health_Refs.ctl" = cluster{"Group_ref":T14, "TE_Temp1_dset":T14, "TE_Outp1_dset":T14, "TE_Temp2_dset":T14, "TE_Outp2_dset":T14, "TE_Temp3_dset":T14, "TE_Outp3_dset":T14, "TimeStamp":T14}
  T22 = typedef "UPS_refs.ctl" = cluster{"Group_ref":T14, "TimeString_dset":T14, "TimeStamp_dset":T14, "V_dset":T14, "A_dset":T14, "Hz_dset":T14, "W_dset":T14, "%_dset":T14}
  T23 = typedef "WeatherRefs.ctl" = cluster{"Group_ref":T14, "TimeString_dset":T14, "TimeStamp_dset ":T14, "WindSpd_dset":T14, "WindGusts_dset":T14, "WindDir_dset":T14, "WindDirSTD_dset":T14, "Temp_dset":T14, "Humidity_dset":T14, "Pressure_dset":T14, "RainRate_dset":T14, "RainFall_dset":T14}
  T24 = typedef "HDF5_AI_refs.ctl" = cluster{"Group_ref":T14, "TimeString_dset":T14, "TimeStamp_dset":T14, "AI0_dset":T14, "AI1_dset":T14, "AI2_dset":T14, "AI3_dset":T14, "AI4_dset":T14, "AI5_dset":T14, "AI6_dset":T14, "AI16_dset":T14, "AI17_dset":T14, "AI18_dset":T14, "AzStdDev_dset":T14, "AI19_dset":T14, "ElStdDev_dset":T14, "BlowerPwr_dset":T14}
  T25 = typedef "HDF5_Filter_refs.ctl" = cluster{"Filter_Group_ref":T14, "TimeStamp_dset":T14, "Filter_dset":T14}
  T26 = typedef "HDF5_ADAM_Refs.ctl" = cluster{"Group_ref":T14, "ADAM_CoPol_dset":T14, "ADAM_XPol_dset":T14, "ADAM_Noise_dset":T14, "ADAM_CalBox_dset":T14, "TimeStamp":T14}
  T27 = typedef "HDF5_Complex_Refs.ctl" = cluster{"Group_ref":T14, "TImeStamp_dset":T14, "PwrSpect_dset":T14, "ISpect_dset":T14, "QSpect_dset":T14}
  T28 = typedef "LogDataClust.ctl" = cluster{"Tone":T29[], "TCData":T31, "AI":T32, "NoiseTrace":cluster{"Target":T12, "NoiseTrace":dbl[]}[], "NoiseInfo":cluster{"Target":T12, "HDF5_NoiseInfo":T33}[], "Disdrom":T34[], "Weath":T37[], "TE":T39, "ADAM":T40, "TimeDomain":T41[]}
  T29 = typedef "ToneLogBuffered.ctl" = cluster{"Count":i32, "CalVal":sgl[], "CalLoc":i32[], "BeacVal":sgl[], "BeacLoc":i32[], "BeacShift":i32[], "Enum":T12, "df":dbl, "PwrSpectr":sgl[][], "ISpectr":sgl[][], "QSpectr":sgl[][], "Time":timestamp[], "SNR":sgl[], "AboveThresh":bool[], "10Hz_PeakVal":dbl[], "Phase":sgl[], "DeltaPhase":dbl[], "Saturat":T30, "10MHz":bool}
  T30 = typedef "SaturationMonitorBuffer.ctl" = cluster{"Meas":bool[], "Stage1":bool[], "Stage4":bool[], "Stage5":bool[], "Stage6":bool[], "Stage7":bool[]}
  T31 = typedef "TC_Data_Structure.ctl" = cluster{"TimeStamp":dbl, "TimeString":string, "TC0_LP1_Hi":dbl, "TC1_LP1_MidHi":dbl, "TC2_LP1_Mid":dbl, "TC3_LP1_LoMid":dbl, "TC4_LP1_Lo":dbl, "TC5_LP2_Hi":dbl, "TC6_LP2_MidHi":dbl, "TC7_LP2_Mid":dbl, "TC8_LP2_LoMid":dbl, "TC9_LP2_Lo":dbl, "TC10_HVAC_Cond_In":dbl, "TC11_HVAC_Cond_Out":dbl, "TC12_Gen_Exhaust":dbl, "TC13_Amb_Inter":dbl, "TC14_Unused":dbl, "TC15_Unused":dbl, "TC16_Unused":dbl, "TC17_Unused":dbl, "TC18_Unused":dbl, "TC19_Unused":dbl, "TC20_Unused":dbl, "TC21_Unused":dbl, "TC22_Unused":dbl, "TC23_Unused":dbl, "TC24_Unused":dbl, "TC25_Unused":dbl, "TC26_Unused":dbl, "TC27_Unused":dbl, "TC28_Unused":dbl, "TC29_Unused":dbl, "TC30_Unused":dbl, "TC31_Unused":dbl}
  T32 = typedef "AI_Clust.ctl" = cluster{"TimeString":string, "Time Stamp":dbl, "AI0_Unused":dbl, "AI1_-5V":dbl, "AI2_+5V":dbl, "AI3_+6V":dbl, "AI4_+12V":dbl, "AI5_+15V":dbl, "AI6_+28V":dbl, "AI7_Unused":dbl, "Ai16_72GHz_CalPower":dbl, "Ai17_84GHz_CalPower":dbl, "Ai18_InclinAz":dbl, "Ai19_InclinEl":dbl, "Ai20_BlowerPwr":dbl, "Ai21_Unused":dbl, "Ai22_Unused":dbl, "Ai23_Unused":dbl, "InclinA_StdDev":dbl, "InclinB_StdDev":dbl, "InclinAz_Unfilt":dbl, "InclinEl_Unfilt":dbl}
  T33 = typedef "HDF5_NoiseInfoClust.ctl" = cluster{"Timestring":string, "Timestamp":dbl, "df":dbl, "Sum":dbl}
  T34 = typedef "DisdrometerData.ctl" = cluster{"Spectrum Data":i16[], "DisdromSummary":T35, "Status":T36}
  T35 = typedef "DisdromterSummaryData.ctl" = cluster{"current time":dbl, "Timestamp":dbl, "Total Rain Rate":dbl, "Liquid Rain Rate":dbl, "Solid Rain Rate":dbl, "Total Rainfall":dbl, "Visibility":dbl, "Radar Reflectivity":dbl, "Max Diameter Hail":dbl, "Measured Particles":i32, "Particle Min Speed":i16, "Particle Max Speed":i16, "Particle Min Diam":i16, "NonHydr Particles":i16, "NonHydr Volume":dbl, "Unkn Particles":i16, "Unkn Volume":dbl, "HydroType":i8}
  T36 = typedef "Disdrometer_Status_Cluster.ctl" = cluster{"Laser":bool, "Signal":bool, "LaserTemp_Analog":bool, "LaserTemp_Digital":bool, "LaserCurrent_Analog":bool, "LaserCurrent_Digital":bool, "SensorSupply":bool, "HeatLaserHead":bool, "HeatReceiverHead":bool, "TempSensor":bool, "HeatSupply":bool, "HeatHousing":bool, "HeatHeads":bool, "HeatCarriers":bool, "OutputLaserPower":bool, "Checksum":bool, "StatusInt":u16}
  T37 = typedef "WeatherDataClust.ctl" = cluster{"TimeString":string, "Timestamp":dbl, "Wind Speed":sgl, "Wind Gusts":sgl, "Wind Dir":sgl, "Wind Dir STD":sgl, "Temperature":sgl, "Humidity":sgl, "Pressure":sgl, "Rain Rate":i16, "Rain Fall":sgl, "Status":T38}
  T38 = typedef "ValidityWeatherClust.ctl" = cluster{"Temp_OutOfBounds":bool, "Temp_IncrSTD":bool, "Temp_Oth":bool, "BarPress_OutOfBounds":bool, "BarPress_IncrSTD":bool, "BarPress_Change":bool, "BarPress_Other":bool, "Humid_OutOfBounds":bool, "Humid_IncrSTD":bool, "Humid_Other":bool, "Wind__Spd_OutOfBounds":bool, "Wind_Dir_OutOfBounds":bool, "RainBuck_OutOfBounds":bool, "RainBuck_Disdrom":bool, "Disdrom_RainBuck":bool, "Placeholder":bool}
  T39 = typedef "TE_Data_Clust.ctl" = cluster{"TimeString":string, "TimeStamp":dbl, "Temp":dbl, "Output":dbl, "Temp 2":dbl, "Output 2":dbl, "Temp 3":dbl, "Output 3":dbl}
  T40 = typedef "HDF5_ADAM_Data.ctl" = cluster{"Timestamp":dbl, "Time string":string, "Fault 1":bool, "Fault 2":bool, "Fault 3":bool, "Fault 4":bool, "Fault 5":bool, "Fault 6":bool, "Value 1":dbl, "Value 2":dbl, "Value 3":dbl, "Value 4":dbl, "Value 5":dbl, "Value 6":dbl}
  T41 = typedef "TimeDomainData.ctl" = cluster{"CalTimeVal":dbl[], "CalTimeCount":u32[], "Enum":T12}
  T42 = typedef "AlarmSettingsClust.ctl" = cluster{"TC13":T43, "AI1":T43, "AI2":T43, "AI3":T43, "AI4":T43, "AI5":T43, "AI6":T43, "AI18":T43, "AI19":T43, "TE1":T43, "TE2":T43, "TE3":T43, "ADAM1":T43, "ADAM2":T43, "ADAM3":T43, "ADAM4":T43, "72CoBeacFreq":T43, "72CoCalFreq":T43, "84CoBeacFreq":T43, "84CoCalFreq":T43, "72Co_CalTonePwr":T43, "72X_CalTonePwr":T43, "84Co_CalTonePwr":T43, "84X_CalTonePwr":T43}
  T43 = typedef "AlarmThresh_OneChan.ctl" = cluster{"Enbl":bool, "ErrsAndWarns":cluster{dbl, dbl, dbl, dbl}}
  T44 = typedef "ErrorStatus.ctl" = cluster{"RX?":bool, "Warn":bool, "Error":bool, "Enabl":bool, "Source":string}
  T45 = typedef "DigOutClust.ctl" = cluster{"Green":bool, "Rx_Yell":bool, "Cx_Yell":bool, "Red":bool, "Source":string}
  T46 = typedef "Saturation_Status_Clust.ctl" = cluster{"84":bool[], "72":bool[]}
  T47 = typedef "HDF5_10HzRefs.ctl" = cluster{"72Co_dset":T14, "84Co_dset":T14, "FileRef":T14}
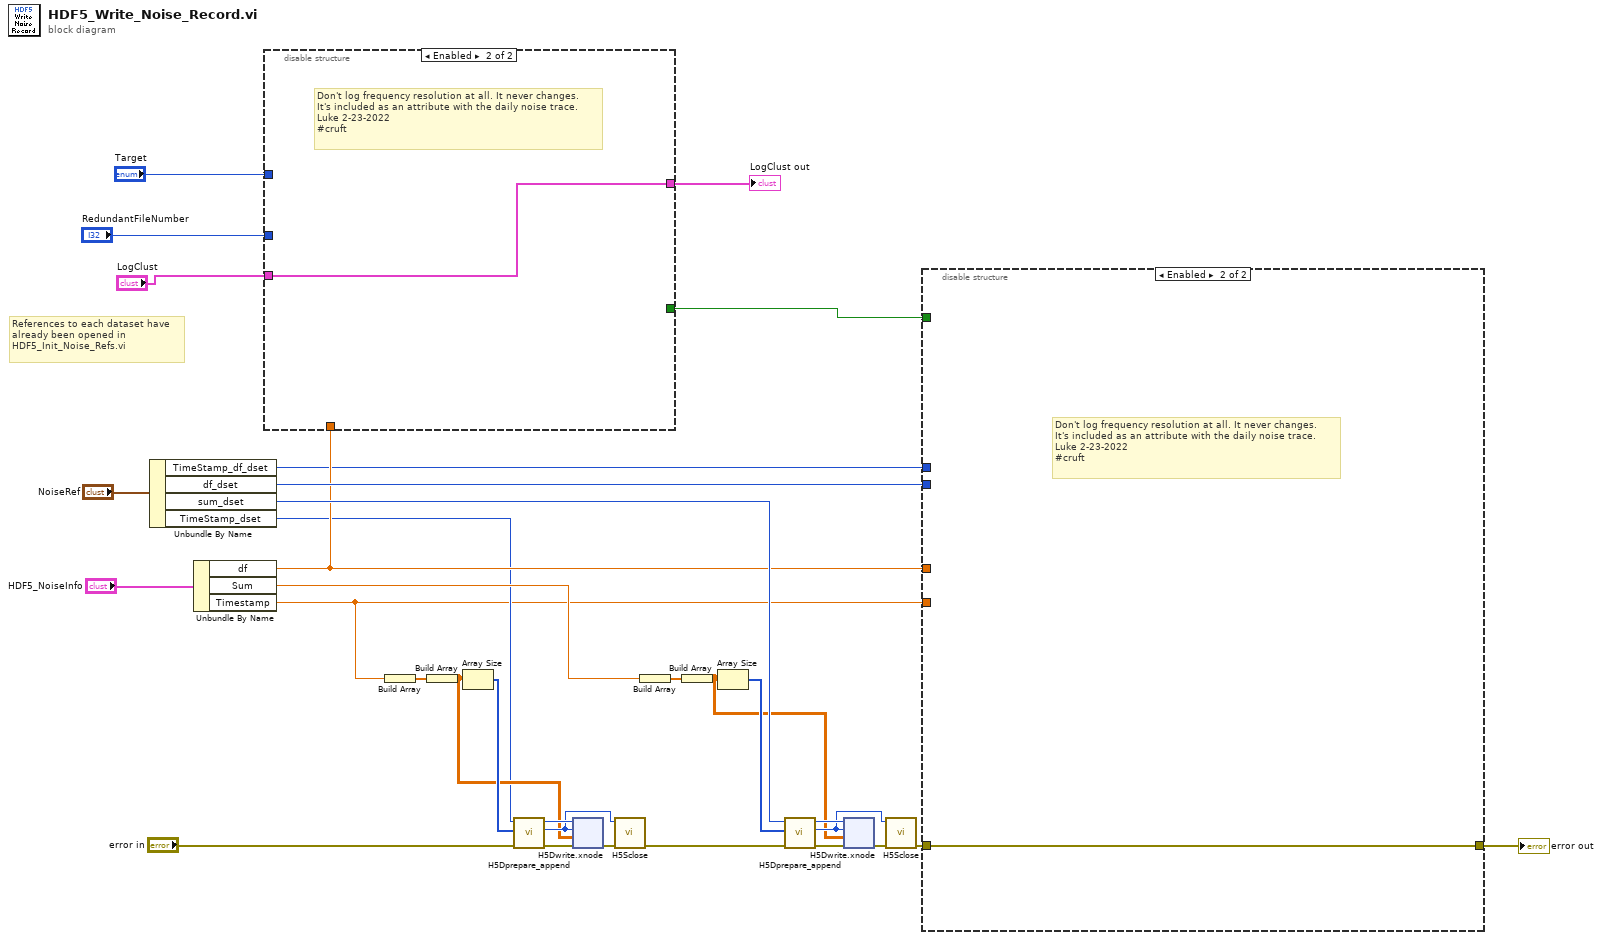
[diagram p0: block diagram]
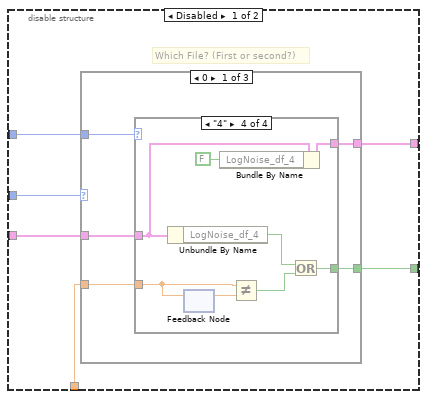
[diagram p2: hidden frame]
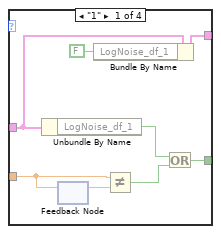
[diagram p3: hidden frame]
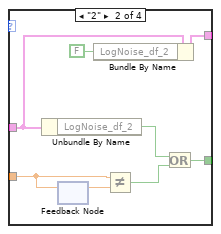
[diagram p4: hidden frame]
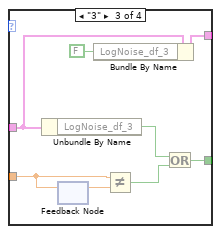
[diagram p5: hidden frame]
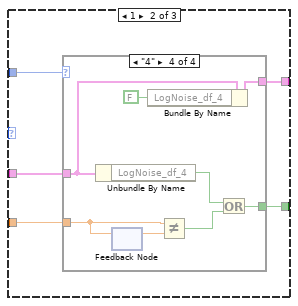
[diagram p6: hidden frame]
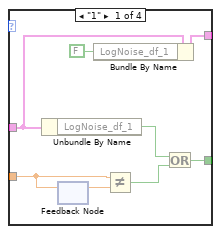
[diagram p7: hidden frame]
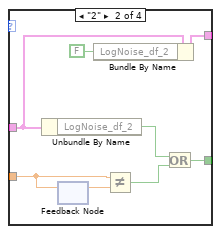
[diagram p8: hidden frame]
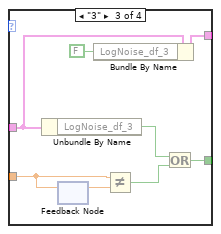
[diagram p9: hidden frame]
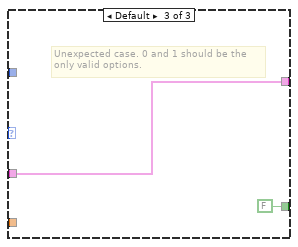
[diagram p10: hidden frame]
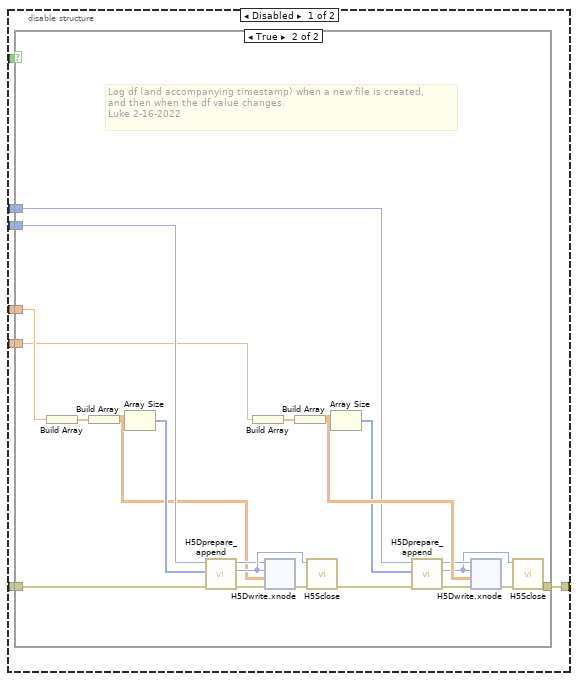
[diagram p11: hidden frame]
diagram:
  # "References to each dataset have \nalready been opened in \nHDF5_Init_Noise_Refs.vi"
  n1 = Unbundle By Name("NoiseRef") -> ("TimeStamp_df_dset"=w5:T14, "df_dset"=w20:T14, "sum_dset"=w19:T14, "TimeStamp_dset"=w6:T14)
  n2 = Unbundle By Name("HDF5_NoiseInfo") -> ("df"=w7:dbl, "Sum"=w16:dbl, "Timestamp"=w4:dbl)
  n3 = disable-structure shown="Enabled" {
    disable-tunnel: "RedundantFileNumber" -> [w38 _]
    disable-tunnel: "Target" -> [w37 _]
    disable-tunnel: "LogClust" -> [w36 w115]
    disable-tunnel: [w35 w115] -> w9
    disable-tunnel: w7 -> [w34 _]
    disable-tunnel: [w33 _] -> w1
    frame Disabled {
      # "Which File? (First or second?)"
      n4 = case shown="0" w38 {
        tunnel: w37 -> [w43 w80 _]
        tunnel: w36 -> [w42 w79 w114]
        tunnel: w34 -> [w41 w78 _]
        tunnel: [w40 w77 FALSE] -> w33
        tunnel: [w39 w76 w114] -> w35
        frame 0 {
          n5 = case shown="\"4\"" w43 {
            tunnel: w42 -> [w46 w54 w62 w70]
            tunnel: w41 -> [w50 w58 w66 w74]
            tunnel: [w47 w55 w63 w71] -> w40
            tunnel: [w45 w53 w61 w69] -> w39
            frame "1" {
              n6 = Unbundle By Name(w46) -> ("LogNoise_df_1"=w49:bool)
              n7 = feedback-in #1(w50) -> ()
              n8 = feedback #1() -> (w51:dbl)  [unwired: 1 in]
              n9 = Bundle By Name(cluster=w46, "LogNoise_df_1"=FALSE) -> (w45:T1)
              n10 = Not Equal?(x=w50, y=w51) -> (x != y?=w48:bool)
              n11 = Or(x=w49, y=w48) -> (x .or. y?=w47:bool)
            }
            frame "2" {
              n12 = Unbundle By Name(w54) -> ("LogNoise_df_2"=w57:bool)
              n13 = feedback-in #2(w58) -> ()
              n14 = feedback #2() -> (w59:dbl)  [unwired: 1 in]
              n15 = Bundle By Name(cluster=w54, "LogNoise_df_2"=FALSE ("LogNoise_df_1")) -> (w53:T1)
              n16 = Not Equal?(x=w58, y=w59) -> (x != y?=w56:bool)
              n17 = Or(x=w57, y=w56) -> (x .or. y?=w55:bool)
            }
            frame "3" {
              n18 = Unbundle By Name(w62) -> ("LogNoise_df_3"=w65:bool)
              n19 = feedback-in #3(w66) -> ()
              n20 = feedback #3() -> (w67:dbl)  [unwired: 1 in]
              n21 = Bundle By Name(cluster=w62, "LogNoise_df_3"=FALSE ("LogNoise_df_1")) -> (w61:T1)
              n22 = Not Equal?(x=w66, y=w67) -> (x != y?=w64:bool)
              n23 = Or(x=w65, y=w64) -> (x .or. y?=w63:bool)
            }
            frame "4" {
              n24 = Unbundle By Name(w70) -> ("LogNoise_df_4"=w73:bool)
              n25 = feedback-in #4(w74) -> ()
              n26 = feedback #4() -> (w75:dbl)  [unwired: 1 in]
              n27 = Bundle By Name(cluster=w70, "LogNoise_df_4"=FALSE ("LogNoise_df_1")) -> (w69:T1)
              n28 = Not Equal?(x=w74, y=w75) -> (x != y?=w72:bool)
              n29 = Or(x=w73, y=w72) -> (x .or. y?=w71:bool)
            }
          }
        }
        frame 1 {
          n30 = case shown="\"4\"" w80 {
            tunnel: w79 -> [w83 w91 w99 w107]
            tunnel: w78 -> [w87 w95 w103 w111]
            tunnel: [w84 w92 w100 w108] -> w77
            tunnel: [w82 w90 w98 w106] -> w76
            frame "1" {
              n31 = Unbundle By Name(w83) -> ("LogNoise_df_1"=w86:bool)
              n32 = feedback-in #5(w87) -> ()
              n33 = feedback #5() -> (w88:dbl)  [unwired: 1 in]
              n34 = Bundle By Name(cluster=w83, "LogNoise_df_1"=FALSE) -> (w82:T1)
              n35 = Not Equal?(x=w87, y=w88) -> (x != y?=w85:bool)
              n36 = Or(x=w86, y=w85) -> (x .or. y?=w84:bool)
            }
            frame "2" {
              n37 = Unbundle By Name(w91) -> ("LogNoise_df_2"=w94:bool)
              n38 = feedback-in #6(w95) -> ()
              n39 = feedback #6() -> (w96:dbl)  [unwired: 1 in]
              n40 = Bundle By Name(cluster=w91, "LogNoise_df_2"=FALSE ("LogNoise_df_1")) -> (w90:T1)
              n41 = Not Equal?(x=w95, y=w96) -> (x != y?=w93:bool)
              n42 = Or(x=w94, y=w93) -> (x .or. y?=w92:bool)
            }
            frame "3" {
              n43 = Unbundle By Name(w99) -> ("LogNoise_df_3"=w102:bool)
              n44 = feedback-in #7(w103) -> ()
              n45 = feedback #7() -> (w104:dbl)  [unwired: 1 in]
              n46 = Bundle By Name(cluster=w99, "LogNoise_df_3"=FALSE ("LogNoise_df_1")) -> (w98:T1)
              n47 = Not Equal?(x=w103, y=w104) -> (x != y?=w101:bool)
              n48 = Or(x=w102, y=w101) -> (x .or. y?=w100:bool)
            }
            frame "4" {
              n49 = Unbundle By Name(w107) -> ("LogNoise_df_4"=w110:bool)
              n50 = feedback-in #8(w111) -> ()
              n51 = feedback #8() -> (w112:dbl)  [unwired: 1 in]
              n52 = Bundle By Name(cluster=w107, "LogNoise_df_4"=FALSE ("LogNoise_df_1")) -> (w106:T1)
              n53 = Not Equal?(x=w111, y=w112) -> (x != y?=w109:bool)
              n54 = Or(x=w110, y=w109) -> (x .or. y?=w108:bool)
            }
          }
        }
        frame Default {
          # "Unexpected case. 0 and 1 should be the \nonly valid options."
        }
      }
    }
    frame Enabled {
      # "Don't log frequency resolution at all. It never changes.\nIt's included as an attribute with the daily noise trace.\nLuke 2-23-2022\n#cruft"
    }
  }
  "LogClust out" <- w9
  n55 = Build Array(w4) -> (w23:dbl[])
  n56 = Build Array(w23) -> (w14:dbl[][])
  n57 = Array Size(array=w14) -> (size(s)=w22:i32[])
  n58 = call <vilib>:"H5Dprepare_append.vi"("error in (no error)"="error in", "append dims"=w22, "dset in"=w6) -> ("error out"=w28:errorcluster, "space out"=w30:T14, "dset out"=w31:T14)  [unwired: 5 in, 1 out]
  n59 = xnode "H5Dwrite.xnode"("error in (no error)"=w28, "data"=w14, "file space"=w30, "ref in"=w31) -> ("error out"=w29:errorcluster)  [unwired: 3 in, 2 out]
  n60 = call <vilib>:"H5Sclose.vi"("error in (no error)"=w29, "space in"=w30) -> ("error out"=w8:errorcluster)  [unwired: 9 in]
  n61 = Build Array(w16) -> (w18:dbl[])
  n62 = Build Array(w18) -> (w15:dbl[][])
  n63 = Array Size(array=w15) -> (size(s)=w17:i32[])
  n64 = call <vilib>:"H5Dprepare_append.vi"("error in (no error)"=w8, "append dims"=w17, "dset in"=w19) -> ("error out"=w24:errorcluster, "space out"=w26:T14, "dset out"=w27:T14)  [unwired: 5 in, 1 out]
  n65 = xnode "H5Dwrite.xnode"("error in (no error)"=w24, "data"=w15, "file space"=w26, "ref in"=w27) -> ("error out"=w25:errorcluster)  [unwired: 3 in, 2 out]
  n66 = call <vilib>:"H5Sclose.vi"("error in (no error)"=w25, "space in"=w26) -> ("error out"=w3:errorcluster)  [unwired: 9 in]
  n67 = disable-structure shown="Enabled" {
    disable-tunnel: w20 -> [w122 _]
    disable-tunnel: w7 -> [w121 _]
    disable-tunnel: w5 -> [w120 _]
    disable-tunnel: w4 -> [w119 _]
    disable-tunnel: w3 -> [w118 w183]
    disable-tunnel: [w117 w183] -> w2
    disable-tunnel: w1 -> [w116 _]
    frame Disabled {
      n68 = case shown="True" w116 {
        tunnel: w122 -> [_ w140]
        tunnel: w121 -> [_ w136]
        tunnel: w120 -> [_ w128]
        tunnel: w119 -> [_ w127]
        tunnel: w118 -> [w123 w126]
        tunnel: [w123 w124] -> w117
        frame False {
        }
        frame True {
          # "Log df (and accompanying timestamp) when a new file is created,\nand then when the df value changes.\nLuke 2-16-2022"
          n69 = Build Array(w136) -> (w139:dbl[])
          n70 = Build Array(w139) -> (w137:dbl[][])
          n71 = Array Size(array=w137) -> (size(s)=w138:i32[])
          n72 = call <vilib>:"H5Dprepare_append.vi"("error in (no error)"=w126, "append dims"=w138, "dset in"=w140) -> ("error out"=w144:errorcluster, "space out"=w142:T14, "dset out"=w141:T14)  [unwired: 5 in, 1 out]
          n73 = Build Array(w127) -> (w133:dbl[])
          n74 = xnode "H5Dwrite.xnode"("error in (no error)"=w144, "data"=w137, "file space"=w142, "ref in"=w141) -> ("error out"=w143:errorcluster)  [unwired: 3 in, 2 out]
          n75 = Build Array(w133) -> (w135:dbl[][])
          n76 = call <vilib>:"H5Sclose.vi"("error in (no error)"=w143, "space in"=w142) -> ("error out"=w125:errorcluster)  [unwired: 9 in]
          n77 = Array Size(array=w135) -> (size(s)=w134:i32[])
          n78 = call <vilib>:"H5Dprepare_append.vi"("error in (no error)"=w125, "append dims"=w134, "dset in"=w128) -> ("error out"=w129:errorcluster, "space out"=w131:T14, "dset out"=w132:T14)  [unwired: 5 in, 1 out]
          n79 = xnode "H5Dwrite.xnode"("error in (no error)"=w129, "data"=w135, "file space"=w131, "ref in"=w132) -> ("error out"=w130:errorcluster)  [unwired: 3 in, 2 out]
          n80 = call <vilib>:"H5Sclose.vi"("error in (no error)"=w130, "space in"=w131) -> ("error out"=w124:errorcluster)  [unwired: 9 in]
        }
      }
    }
    frame Enabled {
      # "Don't log frequency resolution at all. It never changes.\nIt's included as an attribute with the daily noise trace.\nLuke 2-23-2022\n#cruft"
    }
  }
  "error out" <- w2
